vi "IV(H)_2devices_DC_vector_magnet_angle+temperature_sweep_BF_LD-400_K6221_K2182A_PK.vi"() -> ()   [LabVIEW 2016]
uses:
  <vilib>/Math Plots/2D Math Plots/2D Compass/2D Compass XCtrl/2D Compass.xctl
  <vilib>/Math Plots/2D Math Plots/2D Compass/2D Compass Datatype/2D Compass Datatype.lvclass
  <vilib>/Math Plots/2D Math Plots/2D Compass/2D Compass Datatype/Public/Plot Helper (Vector).vi
  Labview Drivers/Keithley 622x LV 2009/Keithley 622x.lvlib
  Labview Drivers/lake_shore_372/Lake Shore 372/Lake Shore 372.lvlib
panel:
  out "Still temperature (K)":dbl=0.747234 min=0.0 max=1000.0 step=1e-05 format="%^.5e"
  out "Still Output (%)":dbl=13.69 min=0.0 max=100.0 step=1e-05 format="%^.5e"
  out "Magnet temperature (K)":dbl=3.7122 min=0.0 max=1000.0 step=1e-05 format="%.5f"
  in  "From 5":dbl[](array[numeric])=[0.0] min=-3000.0 max=3000.0 format="%#.5f"
  in  "To 5":dbl[](array[numeric])=[0.0] min=-3000.0 max=3000.0 format="%#.5g"
  in  "Step 5":dbl[](array[numeric])=[0.001] min=-3000.0 max=3000.0 format="%.5e"
  in  "Still Heater Output (%)":dbl=13.69
  in  "Heater Range (0: Off)":u16(ring)=6 items=["Off", "31.6 uA", "100 uA", "316 uA", "1.00 mA", "3.16 mA", "10.0 mA", "31.6 mA", "100 mA"]
  in  "Output (0: sample heater)":u16(ring) items=["sample heater", "output 1 (warm-up heater) ", "output 2 (analog/still)"]
  in  "Rate(D) (0)":dbl min=0.0 max=2500.0 step=1.0 format="%.6f"
  in  "Reset(I) (20)":dbl=20.0 min=0.0 max=10000.0 step=1.0 format="%.6f"
  in  "Gain(P) (10.000)":dbl=10.0 min=0.001 max=1000.0 step=0.001 format="%.6f"
  out "Set Temperature (K)":dbl=0.9999999999999999 format="%#_13g"
  out "Delay timer (s)":i32=600
  in  "T settling delay (s)":i32=60
  out "Heater Output (%)":dbl=7.0 min=0.0 max=100.0 step=1e-05 format="%^.5e"
  out "Current Temperature (K)":dbl=1.00279 format="%#_13g"
  out "data 2":dbl[](array[numeric])=[0.0, 0.1539956170131437, 179.99925141305565, -5.8e-05, -0.000894677769, 15.42547877586207, 62218.001]
  out "File path 2":path=path "D:/Malli/GeTe/VNM519/027_VNM519_Dev1_DC_IV_baseT_OOP-Y-axis(250_to_-250mT)_1mT_steps_I16-19_V17-18_(K6221_12- K2182_4).dat"
  in  "Measure two devices?":bool
  out "2D Compass":refnum<class "2D Plot Datatype.lvclass">[](xcontrol)
  in  "Number Averaging":i32=1
  in  "Tab Control":enum32{"Device 1", "Device 2"}(tab)
  out "V vs I":cluster{dbl, "Field Reading":dbl}[](graph)=[{0.0, "Field Reading"=-1.52268497e-07}, {2e-07, "Field Reading"=-7.97594228e-08}, {4e-07, "Field Reading"=-2.74494669e-08}, {6e-07, "Field Reading"=2.5999633e-07}, {8e-07, "Field Reading"=6.6863549e-07}, {1e-06, "Field Reading"=9.26042323e-07}, {1.2e-06, "Field Reading"=1.14823021e-06}, {1.4e-06, "Field Reading"=1.4843606e-06}, {1.6e-06, "Field Reading"=1.76714547e-06}, {1.8e-06, "Field Reading"=1.96654487e-06}, {2e-06, "Field Reading"=2.31562332e-06}, {2.2e-06, "Field Reading"=2.42801356e-06}, {2.4e-06, "Field Reading"=2.6657392e-06}, {2.6e-06, "Field Reading"=3.04123176e-06}, {2.8e-06, "Field Reading"=3.30122805e-06}, {3e-06, "Field Reading"=3.42190359e-06}, {3.2e-06, "Field Reading"=3.80050368e-06}, {3.4e-06, "Field Reading"=3.8305433e-06}, {3.6e-06, "Field Reading"=4.18790866e-06}, {3.8e-06, "Field Reading"=4.36969886e-06}, {4e-06, "Field Reading"=4.7099712e-06}, {4.2e-06, "Field Reading"=5.08080239e-06}, {4.4e-06, "Field Reading"=5.22633809e-06}, {4.6e-06, "Field Reading"=5.43764972e-06}, {4.8e-06, "Field Reading"=5.58784671e-06}, {5e-06, "Field Reading"=5.92760266e-06}, {5.2e-06, "Field Reading"=6.16066695e-06}, {5.4e-06, "Field Reading"=6.52631866e-06}, {5.6e-06, "Field Reading"=6.60711428e-06}, {5.8e-06, "Field Reading"=6.8862735e-06}, {6e-06, "Field Reading"=7.20945277e-06}, {6.2e-06, "Field Reading"=7.31976981e-06}, {6.4e-06, "Field Reading"=7.68645747e-06}, {6.6e-06, "Field Reading"=7.9987682e-06}, {6.8e-06, "Field Reading"=8.25462103e-06}, {7e-06, "Field Reading"=8.2913934e-06}, {7.2e-06, "Field Reading"=8.71400919e-06}, {7.4e-06, "Field Reading"=8.98850694e-06}, {7.6e-06, "Field Reading"=9.18531665e-06}, {7.8e-06, "Field Reading"=9.47948819e-06}, {8e-06, "Field Reading"=9.61984449e-06}, {8.2e-06, "Field Reading"=9.91195133e-06}, {8.4e-06, "Field Reading"=1.00347079e-05}, {8.6e-06, "Field Reading"=1.03490855e-05}, {8.8e-06, "Field Reading"=1.06489614e-05}, {9e-06, "Field Reading"=1.08991132e-05}, {9.2e-06, "Field Reading"=1.1134249e-05}, {9.4e-06, "Field Reading"=1.13165569e-05}, {9.6e-06, "Field Reading"=1.15257967e-05}, {9.8e-06, "Field Reading"=1.18443188e-05}, {1e-05, "Field Reading"=1.21214061e-05}, {1.02e-05, "Field Reading"=1.23254667e-05}, {1.04e-05, "Field Reading"=1.26320829e-05}, {1.06e-05, "Field Reading"=1.27895307e-05}, {1.08e-05, "Field Reading"=1.30749049e-05}, {1.1e-05, "Field Reading"=1.32494289e-05}, {1.12e-05, "Field Reading"=1.34664374e-05}, {1.14e-05, "Field Reading"=1.3915992e-05}, {1.16e-05, "Field Reading"=1.40470318e-05}, {1.18e-05, "Field Reading"=1.43101353e-05}, {1.2e-05, "Field Reading"=1.45571832e-05}, {1.22e-05, "Field Reading"=1.46328053e-05}, {1.24e-05, "Field Reading"=1.50393728e-05}, {1.26e-05, "Field Reading"=1.51921593e-05}, {1.28e-05, "Field Reading"=1.54972138e-05}, {1.3e-05, "Field Reading"=1.57333855e-05}, {1.32e-05, "Field Reading"=1.59866486e-05}, {1.34e-05, "Field Reading"=1.6305696e-05}, {1.36e-05, "Field Reading"=1.64346582e-05}, {1.38e-05, "Field Reading"=1.66801526e-05}, {1.4e-05, "Field Reading"=1.69613835e-05}, {1.42e-05, "Field Reading"=1.71208941e-05}, {1.44e-05, "Field Reading"=1.74218058e-05}, {1.46e-05, "Field Reading"=1.76522803e-05}, {1.48e-05, "Field Reading"=1.80106844e-05}, {1.5e-05, "Field Reading"=1.80904442e-05}, {1.52e-05, "Field Reading"=1.83623524e-05}, {1.54e-05, "Field Reading"=1.86627412e-05}, {1.56e-05, "Field Reading"=1.88631763e-05}, {1.58e-05, "Field Reading"=1.90320183e-05}, {1.6e-05, "Field Reading"=1.93800576e-05}, {1.62e-05, "Field Reading"=1.9578939e-05}, {1.64e-05, "Field Reading"=1.97788562e-05}, {1.66e-05, "Field Reading"=2.00880632e-05}, {1.68e-05, "Field Reading"=2.0350131e-05}, {1.7e-05, "Field Reading"=2.05593708e-05}, {1.72e-05, "Field Reading"=2.0896531e-05}, {1.74e-05, "Field Reading"=2.10658909e-05}, {1.76e-05, "Field Reading"=2.11917455e-05}, {1.78e-05, "Field Reading"=2.15387632e-05}, {1.8e-05, "Field Reading"=2.17775246e-05}, {1.82e-05, "Field Reading"=2.19841749e-05}, {1.84e-05, "Field Reading"=2.22824971e-05}, {1.86e-05, "Field Reading"=2.24321761e-05}, {1.88e-05, "Field Reading"=2.27020127e-05}, {1.9e-05, "Field Reading"=2.29822077e-05}, {1.92e-05, "Field Reading"=2.32157907e-05}, {1.94e-05, "Field Reading"=2.3448855e-05}, {1.96e-05, "Field Reading"=2.36135537e-05}, {1.98e-05, "Field Reading"=2.38725181e-05}, {2e-05, "Field Reading"=2.41837884e-05}, {2.02e-05, "Field Reading"=2.43945821e-05}, {2.04e-05, "Field Reading"=2.46193413e-05}, {2.06e-05, "Field Reading"=2.49093766e-05}, {2.08e-05, "Field Reading"=2.51222418e-05}, {2.1e-05, "Field Reading"=2.52900611e-05}, {2.12e-05, "Field Reading"=2.55407347e-05}, {2.14e-05, "Field Reading"=2.58758293e-05}, {2.16e-05, "Field Reading"=2.60860873e-05}, {2.18e-05, "Field Reading"=2.6178795e-05}, {2.2e-05, "Field Reading"=2.6620063e-05}, {2.22e-05, "Field Reading"=2.67676686e-05}, {2.24e-05, "Field Reading"=2.69230447e-05}, {2.26e-05, "Field Reading"=2.72975009e-05}, {2.28e-05, "Field Reading"=2.7582357e-05}, {2.3e-05, "Field Reading"=2.77507011e-05}, {2.32e-05, "Field Reading"=2.80096614e-05}, {2.34e-05, "Field Reading"=2.81696988e-05}, {2.36e-05, "Field Reading"=2.85907685e-05}, {2.38e-05, "Field Reading"=2.87735944e-05}, {2.4e-05, "Field Reading"=2.90294472e-05}, {2.42e-05, "Field Reading"=2.9178615e-05}, {2.44e-05, "Field Reading"=2.96002024e-05}, {2.46e-05, "Field Reading"=2.9786136e-05}, {2.48e-05, "Field Reading"=2.99565396e-05}, {2.6e-05, "Field Reading"=3.14186299e-05}, {2.7e-05, "Field Reading"=3.26751057e-05}, {2.8e-05, "Field Reading"=3.38378258e-05}, {2.9e-05, "Field Reading"=3.52035824e-05}, {3e-05, "Field Reading"=3.63435256e-05}, {3e-05, "Field Reading"=3.63673343e-05}, {1.501e-05, "Field Reading"=1.79573366e-05}, {2e-08, "Field Reading"=-3.87921991e-07}, {0.0, "Field Reading"=-3.45452353e-07}, {-2e-07, "Field Reading"=-3.83778479e-07}, {-4e-07, "Field Reading"=-4.92023888e-07}, {-6e-07, "Field Reading"=-7.5460964e-07}, {-8e-07, "Field Reading"=-1.24196958e-06}, {-1e-06, "Field Reading"=-1.538736e-06}, {-1.2e-06, "Field Reading"=-1.68893191e-06}, {-1.4e-06, "Field Reading"=-2.02972104e-06}, {-1.6e-06, "Field Reading"=-2.24103112e-06}, {-1.8e-06, "Field Reading"=-2.59114291e-06}, {-2e-06, "Field Reading"=-2.7993462e-06}, {-2.2e-06, "Field Reading"=-2.92209253e-06}, {-2.4e-06, "Field Reading"=-3.30068989e-06}, {-2.6e-06, "Field Reading"=-3.44466872e-06}, {-2.8e-06, "Field Reading"=-3.70673454e-06}, {-3e-06, "Field Reading"=-3.97190785e-06}, {-3.2e-06, "Field Reading"=-4.17493005e-06}, {-3.4e-06, "Field Reading"=-4.41472537e-06}, {-3.6e-06, "Field Reading"=-4.66177152e-06}, {-3.8e-06, "Field Reading"=-4.9191763e-06}, {-4e-06, "Field Reading"=-5.20920954e-06}, {-4.2e-06, "Field Reading"=-5.55465984e-06}, {-4.4e-06, "Field Reading"=-5.66652605e-06}, {-4.6e-06, "Field Reading"=-5.96691739e-06}, {-4.8e-06, "Field Reading"=-6.19013923e-06}, {-5e-06, "Field Reading"=-6.40818191e-06}, {-5.2e-06, "Field Reading"=-6.672842e-06}, {-5.4e-06, "Field Reading"=-6.9483736e-06}, {-5.6e-06, "Field Reading"=-7.18713312e-06}, {-5.8e-06, "Field Reading"=-7.36218605e-06}, {-6e-06, "Field Reading"=-7.68329416e-06}, {-6.2e-06, "Field Reading"=-7.86922612e-06}, {-6.4e-06, "Field Reading"=-8.26853861e-06}, {-6.6e-06, "Field Reading"=-8.30634649e-06}, {-6.8e-06, "Field Reading"=-8.59586168e-06}, {-7e-06, "Field Reading"=-9.00657456e-06}, {-7.2e-06, "Field Reading"=-9.14951953e-06}, {-7.4e-06, "Field Reading"=-9.39708366e-06}, {-7.6e-06, "Field Reading"=-9.56643916e-06}, {-7.8e-06, "Field Reading"=-9.81970027e-06}, {-8e-06, "Field Reading"=-1.00263489e-05}, {-8.2e-06, "Field Reading"=-1.02837565e-05}, {-8.4e-06, "Field Reading"=-1.06437086e-05}, {-8.6e-06, "Field Reading"=-1.07623114e-05}, {-8.8e-06, "Field Reading"=-1.09855426e-05}, {-9e-06, "Field Reading"=-1.11694032e-05}, {-9.2e-06, "Field Reading"=-1.15034596e-05}, {-9.4e-06, "Field Reading"=-1.17209848e-05}, {-9.6e-06, "Field Reading"=-1.19462748e-05}, {-9.8e-06, "Field Reading"=-1.21871062e-05}, {-1e-05, "Field Reading"=-1.24362242e-05}, {-1.02e-05, "Field Reading"=-1.26667036e-05}, {-1.04e-05, "Field Reading"=-1.30364964e-05}, {-1.06e-05, "Field Reading"=-1.32317511e-05}, {-1.08e-05, "Field Reading"=-1.35373222e-05}, {-1.1e-05, "Field Reading"=-1.37237724e-05}, {-1.12e-05, "Field Reading"=-1.40371123e-05}, {-1.14e-05, "Field Reading"=-1.42893266e-05}, {-1.16e-05, "Field Reading"=-1.43830695e-05}, {-1.18e-05, "Field Reading"=-1.46358129e-05}, {-1.2e-05, "Field Reading"=-1.50543024e-05}, {-1.22e-05, "Field Reading"=-1.51656546e-05}, {-1.24e-05, "Field Reading"=-1.54468836e-05}, {-1.26e-05, "Field Reading"=-1.56442061e-05}, {-1.28e-05, "Field Reading"=-1.580735e-05}, {-1.3e-05, "Field Reading"=-1.61113673e-05}, {-1.32e-05, "Field Reading"=-1.62418839e-05}, {-1.34e-05, "Field Reading"=-1.6634983e-05}, {-1.36e-05, "Field Reading"=-1.68178077e-05}, {-1.38e-05, "Field Reading"=-1.69198374e-05}, {-1.4e-05, "Field Reading"=-1.7212986e-05}, {-1.42e-05, "Field Reading"=-1.74341367e-05}, {-1.44e-05, "Field Reading"=-1.77231346e-05}, {-1.46e-05, "Field Reading"=-1.78510457e-05}, {-1.48e-05, "Field Reading"=-1.81830304e-05}, {-1.5e-05, "Field Reading"=-1.83668909e-05}, {-1.52e-05, "Field Reading"=-1.86812606e-05}, {-1.54e-05, "Field Reading"=-1.87755215e-05}, {-1.56e-05, "Field Reading"=-1.91867473e-05}, {-1.58e-05, "Field Reading"=-1.92447572e-05}, {-1.6e-05, "Field Reading"=-1.95373802e-05}, {-1.62e-05, "Field Reading"=-1.98776515e-05}, {-1.64e-05, "Field Reading"=-2.01619878e-05}, {-1.66e-05, "Field Reading"=-2.03448124e-05}, {-1.68e-05, "Field Reading"=-2.05985916e-05}, {-1.7e-05, "Field Reading"=-2.09740769e-05}, {-1.72e-05, "Field Reading"=-2.10243148e-05}, {-1.74e-05, "Field Reading"=-2.14578111e-05}, {-1.76e-05, "Field Reading"=-2.17752926e-05}, {-1.78e-05, "Field Reading"=-2.20503063e-05}, {-1.8e-05, "Field Reading"=-2.21507822e-05}, {-1.82e-05, "Field Reading"=-2.23900597e-05}, {-1.84e-05, "Field Reading"=-2.26723233e-05}, {-1.86e-05, "Field Reading"=-2.28976171e-05}, {-1.88e-05, "Field Reading"=-2.31016762e-05}, {-1.9e-05, "Field Reading"=-2.34289957e-05}, {-1.92e-05, "Field Reading"=-2.37117782e-05}, {-1.94e-05, "Field Reading"=-2.40458343e-05}, {-1.96e-05, "Field Reading"=-2.40541191e-05}, {-1.98e-05, "Field Reading"=-2.44544686e-05}, {-2e-05, "Field Reading"=-2.46621531e-05}, {-2.02e-05, "Field Reading"=-2.49703066e-05}, {-2.04e-05, "Field Reading"=-2.5097714e-05}, {-2.06e-05, "Field Reading"=-2.54835617e-05}, {-2.08e-05, "Field Reading"=-2.55648796e-05}, {-2.1e-05, "Field Reading"=-2.58497336e-05}, {-2.12e-05, "Field Reading"=-2.60413627e-05}, {-2.14e-05, "Field Reading"=-2.64365387e-05}, {-2.16e-05, "Field Reading"=-2.67032657e-05}, {-2.18e-05, "Field Reading"=-2.68964486e-05}, {-2.2e-05, "Field Reading"=-2.71341792e-05}, {-2.22e-05, "Field Reading"=-2.72719451e-05}, {-2.24e-05, "Field Reading"=-2.75303855e-05}, {-2.26e-05, "Field Reading"=-2.79266128e-05}, {-2.28e-05, "Field Reading"=-2.81301542e-05}, {-2.3e-05, "Field Reading"=-2.83901486e-05}, {-2.32e-05, "Field Reading"=-2.84232953e-05}, {-2.34e-05, "Field Reading"=-2.87630526e-05}, {-2.36e-05, "Field Reading"=-2.91333634e-05}, {-2.38e-05, "Field Reading"=-2.9317224e-05}, {-2.4e-05, "Field Reading"=-2.96481828e-05}, {-2.42e-05, "Field Reading"=-2.98304898e-05}, {-2.44e-05, "Field Reading"=-2.99692916e-05}, {-2.46e-05, "Field Reading"=-3.02660647e-05}, {-2.48e-05, "Field Reading"=-3.04944663e-05}, {-2.6e-05, "Field Reading"=-3.20653099e-05}, {-2.7e-05, "Field Reading"=-3.32523697e-05}, {-2.8e-05, "Field Reading"=-3.44534201e-05}, {-2.9e-05, "Field Reading"=-3.56938321e-05}, {-3e-05, "Field Reading"=-3.69958442e-05}, {-3e-05, "Field Reading"=-3.70222579e-05}, {-1.501e-05, "Field Reading"=-1.84243803e-05}, {-2e-08, "Field Reading"=-2.59477872e-07}]
  in  "File name 1":string="011_31-05-2022_DevB4_DC_IV(H)_baseT_[5_to-5mT]_30uT_steps_(0_deg)_I_10-36_V_12-37_100nA_steps"
  in  "From 3":dbl[](array[numeric])=[0.0, 2e-05, 0.0, -2e-05] min=-3000.0 max=3000.0 format="%.1e"
  in  "To 3":dbl[](array[numeric])=[2e-05, 0.0, -2e-05, 0.0] min=-3000.0 max=3000.0 format="%.1e"
  in  "Step 3":dbl[](array[numeric])=[2e-08, 9.99e-06, 2e-08, 9.99e-06] min=-3000.0 max=3000.0 format="%.1e"
  in  "Current source K6221 VISA Device 1":refnum<visa-resource-name>="GPIB0::13::INSTR"
  in  "Nanovoltmeter 2182a VISA Device1":refnum<visa-resource-name>="GPIB0::7::INSTR"
  in  "wait (ms)":u32=50
  in  "Set Compliance voltage (V)":dbl=2.0 min=0.0 step=0.1 format="%_3f"
  out "Resistance (ohm)":dbl=12.9738936 format="%#_13g"
  out "Time (s)":dbl=151861.951 format="%#_13g"
  out "Iset (A)":dbl=-2e-08
  out "Vmeas (V)":dbl=-2.59477872e-07
  in  "File name 2":string="040_31-05-2023_DevB3_DC_IV(A)_baseT_12mT_(0-360deg)_5deg_steps_I_10-38_V_12-31_"
  in  "Current source K6221 VISA Device 2":refnum<visa-resource-name>="GPIB0::13::INSTR"
  in  "Nanovoltmeter 2182a VISA Device 2":refnum<visa-resource-name>="GPIB0::7::INSTR"
  in  "Set Compliance voltage (V) 2":dbl=2.0 min=0.0 step=0.1 format="%_3f"
  in  "wait (ms) 2":u32=50
  in  "To 4":dbl[](array[numeric])=[1e-05, 3e-05, -1e-05, -0.0001, 0.0] min=-3000.0 max=3000.0 format="%.1e"
  in  "From 4":dbl[](array[numeric])=[0.0, 1.1e-05, 3e-05, 0.0, -0.0001] min=-3000.0 max=3000.0 format="%.1e"
  in  "Step 4":dbl[](array[numeric])=[2e-07, 1e-06, 0.0, 5e-07, 9.9e-05] min=-3000.0 max=3000.0 format="%.1e"
  out "V vs I 2":cluster{dbl, "Field Reading":dbl}[](graph)=[{0.0, "Field Reading"=1.05982577e-07}, {5e-07, "Field Reading"=1.23902621e-07}, {1e-06, "Field Reading"=4.09598972e-08}, {1.5e-06, "Field Reading"=7.78233302e-08}, {2e-06, "Field Reading"=7.52633791e-08}, {2.5e-06, "Field Reading"=9.9839001e-08}, {3e-06, "Field Reading"=6.70715052e-08}, {3.5e-06, "Field Reading"=6.34878296e-08}, {4e-06, "Field Reading"=1.95069789e-07}, {4.5e-06, "Field Reading"=1.48733775e-06}, {5e-06, "Field Reading"=3.68225755e-06}, {5.5e-06, "Field Reading"=7.0056209e-06}, {6e-06, "Field Reading"=1.131355e-05}, {6.5e-06, "Field Reading"=1.67191983e-05}, {7e-06, "Field Reading"=2.2852904e-05}, {7.5e-06, "Field Reading"=2.94079847e-05}, {8e-06, "Field Reading"=3.63951874e-05}, {8.5e-06, "Field Reading"=4.35057808e-05}, {9e-06, "Field Reading"=5.09056291e-05}, {9.5e-06, "Field Reading"=5.82773365e-05}, {1e-05, "Field Reading"=6.58016184e-05}, {1.05e-05, "Field Reading"=7.33770992e-05}, {1.1e-05, "Field Reading"=8.09648681e-05}, {1.15e-05, "Field Reading"=8.87364392e-05}, {1.2e-05, "Field Reading"=9.64209746e-05}, {1.25e-05, "Field Reading"=0.000104230437}, {1.3e-05, "Field Reading"=0.000112046003}, {1.35e-05, "Field Reading"=0.000119815015}, {1.4e-05, "Field Reading"=0.000127742783}, {1.45e-05, "Field Reading"=0.000135573235}, {1.5e-05, "Field Reading"=0.000143516327}, {1.55e-05, "Field Reading"=0.000151494156}, {1.6e-05, "Field Reading"=0.000159501242}, {1.65e-05, "Field Reading"=0.000167343466}, {1.7e-05, "Field Reading"=0.000175483152}, {1.75e-05, "Field Reading"=0.000183456446}, {1.8e-05, "Field Reading"=0.000191661699}, {1.85e-05, "Field Reading"=0.000199612466}, {1.9e-05, "Field Reading"=0.000207719848}, {1.95e-05, "Field Reading"=0.000215802195}, {2e-05, "Field Reading"=0.00022388403}, {2.05e-05, "Field Reading"=0.000232062763}, {2.1e-05, "Field Reading"=0.000240102107}, {2.15e-05, "Field Reading"=0.000247269011}, {2.2e-05, "Field Reading"=0.000255929973}, {2.25e-05, "Field Reading"=0.000264142372}, {2.3e-05, "Field Reading"=0.000272170452}, {2.35e-05, "Field Reading"=0.000280406012}, {2.4e-05, "Field Reading"=0.000288539055}, {2.45e-05, "Field Reading"=0.000296639977}, {2.5e-05, "Field Reading"=0.000304956829}, {2.55e-05, "Field Reading"=0.000312984916}, {2.6e-05, "Field Reading"=0.000321277684}, {2.65e-05, "Field Reading"=0.000329427113}, {2.7e-05, "Field Reading"=0.00033774076}, {2.75e-05, "Field Reading"=0.000346032008}, {2.8e-05, "Field Reading"=0.000354167609}, {2.85e-05, "Field Reading"=0.000362498087}, {2.9e-05, "Field Reading"=0.000370754002}, {2.95e-05, "Field Reading"=0.000379070387}, {3e-05, "Field Reading"=0.000387405662}, {3.05e-05, "Field Reading"=0.000395624202}, {3.1e-05, "Field Reading"=0.000403926088}, {3.15e-05, "Field Reading"=0.00041243339}, {3.2e-05, "Field Reading"=0.000420845302}, {3.25e-05, "Field Reading"=0.000429363875}, {3.3e-05, "Field Reading"=0.000437565523}, {3.35e-05, "Field Reading"=0.000446109155}, {3.4e-05, "Field Reading"=0.000454533008}, {3.45e-05, "Field Reading"=0.000463127356}, {3.5e-05, "Field Reading"=0.000471630056}, {3.55e-05, "Field Reading"=0.000479936662}, {3.6e-05, "Field Reading"=0.000488525981}, {3.65e-05, "Field Reading"=0.000497198664}, {3.7e-05, "Field Reading"=0.000505853053}, {3.75e-05, "Field Reading"=0.000514436643}, {3.8e-05, "Field Reading"=0.000522915273}, {3.85e-05, "Field Reading"=0.000531648928}, {3.9e-05, "Field Reading"=0.000540244293}, {3.95e-05, "Field Reading"=0.000548950249}, {4e-05, "Field Reading"=0.000557677924}, {4.05e-05, "Field Reading"=0.000566248716}, {4.1e-05, "Field Reading"=0.000574937679}, {4.15e-05, "Field Reading"=0.000583695347}, {4.2e-05, "Field Reading"=0.000592494999}, {4.25e-05, "Field Reading"=0.000601192661}, {4.3e-05, "Field Reading"=0.000609976951}, {4.35e-05, "Field Reading"=0.000618619419}, {4.4e-05, "Field Reading"=0.000627518275}, {4.45e-05, "Field Reading"=0.000636379362}, {4.5e-05, "Field Reading"=0.000644912509}, {4.55e-05, "Field Reading"=0.00065393999}, {4.6e-05, "Field Reading"=0.000662870466}, {4.65e-05, "Field Reading"=0.000671738209}, {4.7e-05, "Field Reading"=0.000680896763}, {4.75e-05, "Field Reading"=0.000689596876}, {4.8e-05, "Field Reading"=0.000698582898}, {4.85e-05, "Field Reading"=0.000707876118}, {4.9e-05, "Field Reading"=0.00071700519}, {4.95e-05, "Field Reading"=0.00072625694}, {5e-05, "Field Reading"=0.000735252693}, {5.05e-05, "Field Reading"=0.000744563505}, {5.1e-05, "Field Reading"=0.000753877714}, {5.15e-05, "Field Reading"=0.000763235462}, {5.2e-05, "Field Reading"=0.000772666405}, {5.25e-05, "Field Reading"=0.000781939653}, {5.3e-05, "Field Reading"=0.00079146705}, {5.35e-05, "Field Reading"=0.000801081283}, {5.4e-05, "Field Reading"=0.000810671964}, {5.45e-05, "Field Reading"=0.000820330099}, {5.5e-05, "Field Reading"=0.000830001161}, {5.55e-05, "Field Reading"=0.000839830429}, {5.6e-05, "Field Reading"=0.000849894446}, {5.65e-05, "Field Reading"=0.000859963842}, {5.7e-05, "Field Reading"=0.00087027569}, {5.75e-05, "Field Reading"=0.000880684023}, {5.8e-05, "Field Reading"=0.000891300225}, {5.85e-05, "Field Reading"=0.000901884572}, {5.9e-05, "Field Reading"=0.00091264413}, {5.95e-05, "Field Reading"=0.000923292586}, {6e-05, "Field Reading"=0.000933904184}, {6.05e-05, "Field Reading"=0.000944740541}, {6.1e-05, "Field Reading"=0.000955724863}, {6.15e-05, "Field Reading"=0.000966541693}, {6.2e-05, "Field Reading"=0.000977790203}, {6.25e-05, "Field Reading"=0.0009887668}, {6.3e-05, "Field Reading"=0.00100003886}, {6.35e-05, "Field Reading"=0.00101126331}, {6.4e-05, "Field Reading"=0.00102284095}, {6.45e-05, "Field Reading"=0.00103437413}, {6.5e-05, "Field Reading"=0.00104578697}, {6.55e-05, "Field Reading"=0.00105781627}, {6.6e-05, "Field Reading"=0.00106970781}, {6.65e-05, "Field Reading"=0.00108158658}, {6.7e-05, "Field Reading"=0.00109345152}, {6.75e-05, "Field Reading"=0.00110520407}, {6.8e-05, "Field Reading"=0.00111705365}, {6.85e-05, "Field Reading"=0.00112896007}, {6.9e-05, "Field Reading"=0.00114097245}, {6.95e-05, "Field Reading"=0.00115300225}, {7e-05, "Field Reading"=0.00116490713}, {7.05e-05, "Field Reading"=0.00117701585}, {7.1e-05, "Field Reading"=0.0011890902}, {7.15e-05, "Field Reading"=0.00120116737}, {7.2e-05, "Field Reading"=0.00121302054}, {7.25e-05, "Field Reading"=0.00122527818}, {7.3e-05, "Field Reading"=0.00123750597}, {7.35e-05, "Field Reading"=0.00124952144}, {7.4e-05, "Field Reading"=0.00126179393}, {7.45e-05, "Field Reading"=0.00127385138}, {7.5e-05, "Field Reading"=0.00128607011}, {7.55e-05, "Field Reading"=0.00129831901}, {7.6e-05, "Field Reading"=0.00131059815}, {7.65e-05, "Field Reading"=0.00132285322}, {7.7e-05, "Field Reading"=0.00133496366}, {7.75e-05, "Field Reading"=0.00134726123}, {7.8e-05, "Field Reading"=0.00135956111}, {7.85e-05, "Field Reading"=0.00137195033}, {7.9e-05, "Field Reading"=0.00138423407}, {7.95e-05, "Field Reading"=0.00139647286}, {8e-05, "Field Reading"=0.00140887898}, {8.05e-05, "Field Reading"=0.00142125669}, {8.1e-05, "Field Reading"=0.00143369762}, {8.15e-05, "Field Reading"=0.00144604179}, {8.2e-05, "Field Reading"=0.00145820055}, {8.25e-05, "Field Reading"=0.0014708299}, {8.3e-05, "Field Reading"=0.001483259}, {8.35e-05, "Field Reading"=0.00149571273}, {8.4e-05, "Field Reading"=0.00150827449}, {8.45e-05, "Field Reading"=0.00152058173}, {8.5e-05, "Field Reading"=0.00153315169}, {8.55e-05, "Field Reading"=0.00154567403}, {8.6e-05, "Field Reading"=0.00155821094}, {8.65e-05, "Field Reading"=0.00157085359}, {8.7e-05, "Field Reading"=0.00158327521}, {8.75e-05, "Field Reading"=0.00159591991}, {8.8e-05, "Field Reading"=0.00160856665}, {8.85e-05, "Field Reading"=0.00162121374}, {8.9e-05, "Field Reading"=0.00163385997}, {8.95e-05, "Field Reading"=0.00164634288}, {9e-05, "Field Reading"=0.00165906267}, {9.05e-05, "Field Reading"=0.00167177904}, {9.1e-05, "Field Reading"=0.00168450438}, {9.15e-05, "Field Reading"=0.00169730779}, {9.2e-05, "Field Reading"=0.00170982705}, {9.25e-05, "Field Reading"=0.00172262613}, {9.3e-05, "Field Reading"=0.00173539114}, {9.35e-05, "Field Reading"=0.00174822988}, {9.4e-05, "Field Reading"=0.00176107221}, {9.45e-05, "Field Reading"=0.00177372408}, {9.5e-05, "Field Reading"=0.00178659463}, {9.55e-05, "Field Reading"=0.00179942159}, {9.6e-05, "Field Reading"=0.00181213335}, {9.65e-05, "Field Reading"=0.00182507038}, {9.7e-05, "Field Reading"=0.00183795264}, {9.75e-05, "Field Reading"=0.00185079437}, {9.8e-05, "Field Reading"=0.0018638159}, {9.85e-05, "Field Reading"=0.00187644421}, {9.9e-05, "Field Reading"=0.0018893681}, {9.95e-05, "Field Reading"=0.001902598}, {0.0001, "Field Reading"=0.00191566643}, {0.0001, "Field Reading"=0.00191578214}, {1e-06, "Field Reading"=1.04959382e-07}, {0.0, "Field Reading"=6.2978119e-08}, {-5e-07, "Field Reading"=7.37299411e-08}, {-1e-06, "Field Reading"=7.32183306e-08}, {-1.5e-06, "Field Reading"=9.8305911e-08}, {-2e-06, "Field Reading"=9.8305911e-08}, {-2.5e-06, "Field Reading"=-9.212857e-09}, {-3e-06, "Field Reading"=7.52657514e-08}, {-3.5e-06, "Field Reading"=-2.29881222e-07}, {-4e-06, "Field Reading"=-9.66638942e-07}, {-4.5e-06, "Field Reading"=-2.71867509e-06}, {-5e-06, "Field Reading"=-5.44042382e-06}, {-5.5e-06, "Field Reading"=-9.24299578e-06}, {-6e-06, "Field Reading"=-1.39195329e-05}, {-6.5e-06, "Field Reading"=-1.93947706e-05}, {-7e-06, "Field Reading"=-2.53845658e-05}, {-7.5e-06, "Field Reading"=-3.17772987e-05}, {-8e-06, "Field Reading"=-3.85647725e-05}, {-8.5e-06, "Field Reading"=-4.54935603e-05}, {-9e-06, "Field Reading"=-5.25713378e-05}, {-9.5e-06, "Field Reading"=-5.9848778e-05}, {-1e-05, "Field Reading"=-6.72593486e-05}, {-1.05e-05, "Field Reading"=-7.46959979e-05}, {-1.1e-05, "Field Reading"=-8.22145956e-05}, {-1.15e-05, "Field Reading"=-8.98888387e-05}, {-1.2e-05, "Field Reading"=-9.7508345e-05}, {-1.25e-05, "Field Reading"=-0.000105279358}, {-1.3e-05, "Field Reading"=-0.000112994564}, {-1.35e-05, "Field Reading"=-0.000120810121}, {-1.4e-05, "Field Reading"=-0.000128620045}, {-1.45e-05, "Field Reading"=-0.00013646688}, {-1.5e-05, "Field Reading"=-0.000144369477}, {-1.55e-05, "Field Reading"=-0.000152356042}, {-1.6e-05, "Field Reading"=-0.00016028334}, {-1.65e-05, "Field Reading"=-0.000168222807}, {-1.7e-05, "Field Reading"=-0.000176283573}, {-1.75e-05, "Field Reading"=-0.000184271677}, {-1.8e-05, "Field Reading"=-0.000192294085}, {-1.85e-05, "Field Reading"=-0.000200345666}, {-1.9e-05, "Field Reading"=-0.00020833633}, {-1.95e-05, "Field Reading"=-0.000216423693}, {-2e-05, "Field Reading"=-0.000224573584}, {-2.05e-05, "Field Reading"=-0.000232658964}, {-2.1e-05, "Field Reading"=-0.000240789835}, {-2.15e-05, "Field Reading"=-0.00024942458}, {-2.2e-05, "Field Reading"=-0.000257524758}, {-2.25e-05, "Field Reading"=-0.000265682837}, {-2.3e-05, "Field Reading"=-0.000273921299}, {-2.35e-05, "Field Reading"=-0.000281918732}, {-2.4e-05, "Field Reading"=-0.000290019983}, {-2.45e-05, "Field Reading"=-0.000298346441}, {-2.5e-05, "Field Reading"=-0.000306562888}, {-2.55e-05, "Field Reading"=-0.000314745032}, {-2.6e-05, "Field Reading"=-0.000322866101}, {-2.65e-05, "Field Reading"=-0.000331147056}, {-2.7e-05, "Field Reading"=-0.000339239598}, {-2.75e-05, "Field Reading"=-0.000347604575}, {-2.8e-05, "Field Reading"=-0.000355902938}, {-2.85e-05, "Field Reading"=-0.000364053667}, {-2.9e-05, "Field Reading"=-0.000372274716}, {-2.95e-05, "Field Reading"=-0.000380721042}, {-3e-05, "Field Reading"=-0.000389052226}, {-3.05e-05, "Field Reading"=-0.000397248701}, {-3.1e-05, "Field Reading"=-0.000405627052}, {-3.15e-05, "Field Reading"=-0.000414022694}, {-3.2e-05, "Field Reading"=-0.000422452566}, {-3.25e-05, "Field Reading"=-0.000430871246}, {-3.3e-05, "Field Reading"=-0.000439115251}, {-3.35e-05, "Field Reading"=-0.000447710054}, {-3.4e-05, "Field Reading"=-0.000456261339}, {-3.45e-05, "Field Reading"=-0.000464751635}, {-3.5e-05, "Field Reading"=-0.000473286534}, {-3.55e-05, "Field Reading"=-0.00048171494}, {-3.6e-05, "Field Reading"=-0.000490283148}, {-3.65e-05, "Field Reading"=-0.000498827776}, {-3.7e-05, "Field Reading"=-0.000507439986}, {-3.75e-05, "Field Reading"=-0.000516045781}, {-3.8e-05, "Field Reading"=-0.0005246155}, {-3.85e-05, "Field Reading"=-0.000533221482}, {-3.9e-05, "Field Reading"=-0.000541909479}, {-3.95e-05, "Field Reading"=-0.000550577507}, {-4e-05, "Field Reading"=-0.000559311386}, {-4.05e-05, "Field Reading"=-0.000567846814}, {-4.1e-05, "Field Reading"=-0.00057664276}, {-4.15e-05, "Field Reading"=-0.000585338952}, {-4.2e-05, "Field Reading"=-0.000594088391}, {-4.25e-05, "Field Reading"=-0.00060273111}, {-4.3e-05, "Field Reading"=-0.000611546081}, {-4.35e-05, "Field Reading"=-0.00062030934}, {-4.4e-05, "Field Reading"=-0.000629159621}, {-4.45e-05, "Field Reading"=-0.0006379664}, {-4.5e-05, "Field Reading"=-0.000646666684}, {-4.55e-05, "Field Reading"=-0.000655509687}, {-4.6e-05, "Field Reading"=-0.000664396847}, {-4.65e-05, "Field Reading"=-0.000673287336}, {-4.7e-05, "Field Reading"=-0.000682299425}, {-4.75e-05, "Field Reading"=-0.000691233691}, {-4.8e-05, "Field Reading"=-0.000700295086}, {-4.85e-05, "Field Reading"=-0.00070939524}, {-4.9e-05, "Field Reading"=-0.000718437027}, {-4.95e-05, "Field Reading"=-0.000727632333}, {-5e-05, "Field Reading"=-0.000736695622}, {-5.05e-05, "Field Reading"=-0.000746025716}, {-5.1e-05, "Field Reading"=-0.000755243116}, {-5.15e-05, "Field Reading"=-0.000764786655}, {-5.2e-05, "Field Reading"=-0.000774240444}, {-5.25e-05, "Field Reading"=-0.000783658543}, {-5.3e-05, "Field Reading"=-0.000793342878}, {-5.35e-05, "Field Reading"=-0.000803049948}, {-5.4e-05, "Field Reading"=-0.000812865349}, {-5.45e-05, "Field Reading"=-0.000822671023}, {-5.5e-05, "Field Reading"=-0.000832792343}, {-5.55e-05, "Field Reading"=-0.000842879097}, {-5.6e-05, "Field Reading"=-0.000853268375}, {-5.65e-05, "Field Reading"=-0.000863553781}, {-5.7e-05, "Field Reading"=-0.00087382946}, {-5.75e-05, "Field Reading"=-0.000884019633}, {-5.8e-05, "Field Reading"=-0.000894677769}]
  out "Vmeas (V) 2":dbl=-0.000894677769
  out "Resistance (ohm) 2":dbl=15.42547877586207 format="%#_13g"
  out "Iset (A) 2":dbl=-5.8e-05
  out "Magnetic Field Vector Angle":dbl=284.9997059221995 format="%#_13g"
  out "Magnetic Field Vector magnitude (T)":dbl=0.11799861557435369 format="%#_13g"
  in  "From 2":dbl[](array[numeric])=[0.005] min=-3000.0 max=3000.0 format="%#.5f"
  in  "To 2":dbl[](array[numeric])=[-0.005] min=-3000.0 max=3000.0 format="%#.5g"
  in  "Step 2":dbl[](array[numeric])=[3e-05] min=-3000.0 max=3000.0 format="%.5e"
  in  "Wait time after each sweep(min)":dbl=0.1 format="%#_13g"
  out "Z-axis Magnetic Field (T)":string="-0.113978067\r\n"
  in  "Y-axis Field ramp rate (T/min)":string="0.0005"
  in  "Z-axis Field ramp rate (T/min)":string="0.0005"
  out "Z-axis (90 deg)":dbl(slide)=-0.113978067 scale=0.0..3.0
  out "Y-Axis (0deg)":dbl(slide)=0.030539704 scale=0.0..3.0
  out "Y-axis Magnetic Field (T)":string="0.030539704\r\n"
  in  "Magnet IP Address Z-axis":string="169.254.207.70"
  in  "Magnet IP Address Y-axis":string="169.254.67.34"
  in  "Magnetic field stabilization time (s)":dbl=1.0 format="%#_13g"
  in  "Step":dbl[](array[numeric])=[0.001] min=-3000.0 max=3000.0 format="%.4g"
  in  "To":dbl[](array[numeric])=[0.0] min=-3000.0 max=3000.0 format="%.4f"
  in  "From":dbl[](array[numeric])=[0.0] min=-3000.0 max=3000.0 format="%.4f"
  in  "Folder":path=path "D:/Pranava/Data/PtTe2/31-05-2022/001/Round8_IP/after warmup"
  out "data":dbl[](array[numeric])=[1.00279, 0.11799861557435369, 284.9997059221995, -2e-08, -2.59477872e-07, 12.9738936, 151861.951]
  out "File path 1":path=path "D:/Pranava/Data/PtTe2/31-05-2022/001/Round8_IP/after warmup/011_31-05-2022_DevB4_DC_IV(H)_baseT_[5_to-5mT]_30uT_steps_(0_deg)_I_10-36_V_12-37_100nA_steps.dat"
  # "11.5% corresponds to 7mW\n13.69% corresponds to 10mW\nSet to 0 if you want to use at 1K"
  # "[Must be less than 0.05]"
  # "It is important that there is enough time for the magnet to cool down after each sweep (Typically 15-20 min)"
  # "Configure Temperature (K)"
  # "Configure Field magnitude (T)"
  # "Configure Field Angle (deg)"
  # "Z-Axis: In-plane (90 deg)\nY-axis: Out-of-plane (0 deg)"
  # ".dat"
  # "Configure current sweep 1 (A)"
  # ".dat"
  # "Configure current sweep 2 (A)"
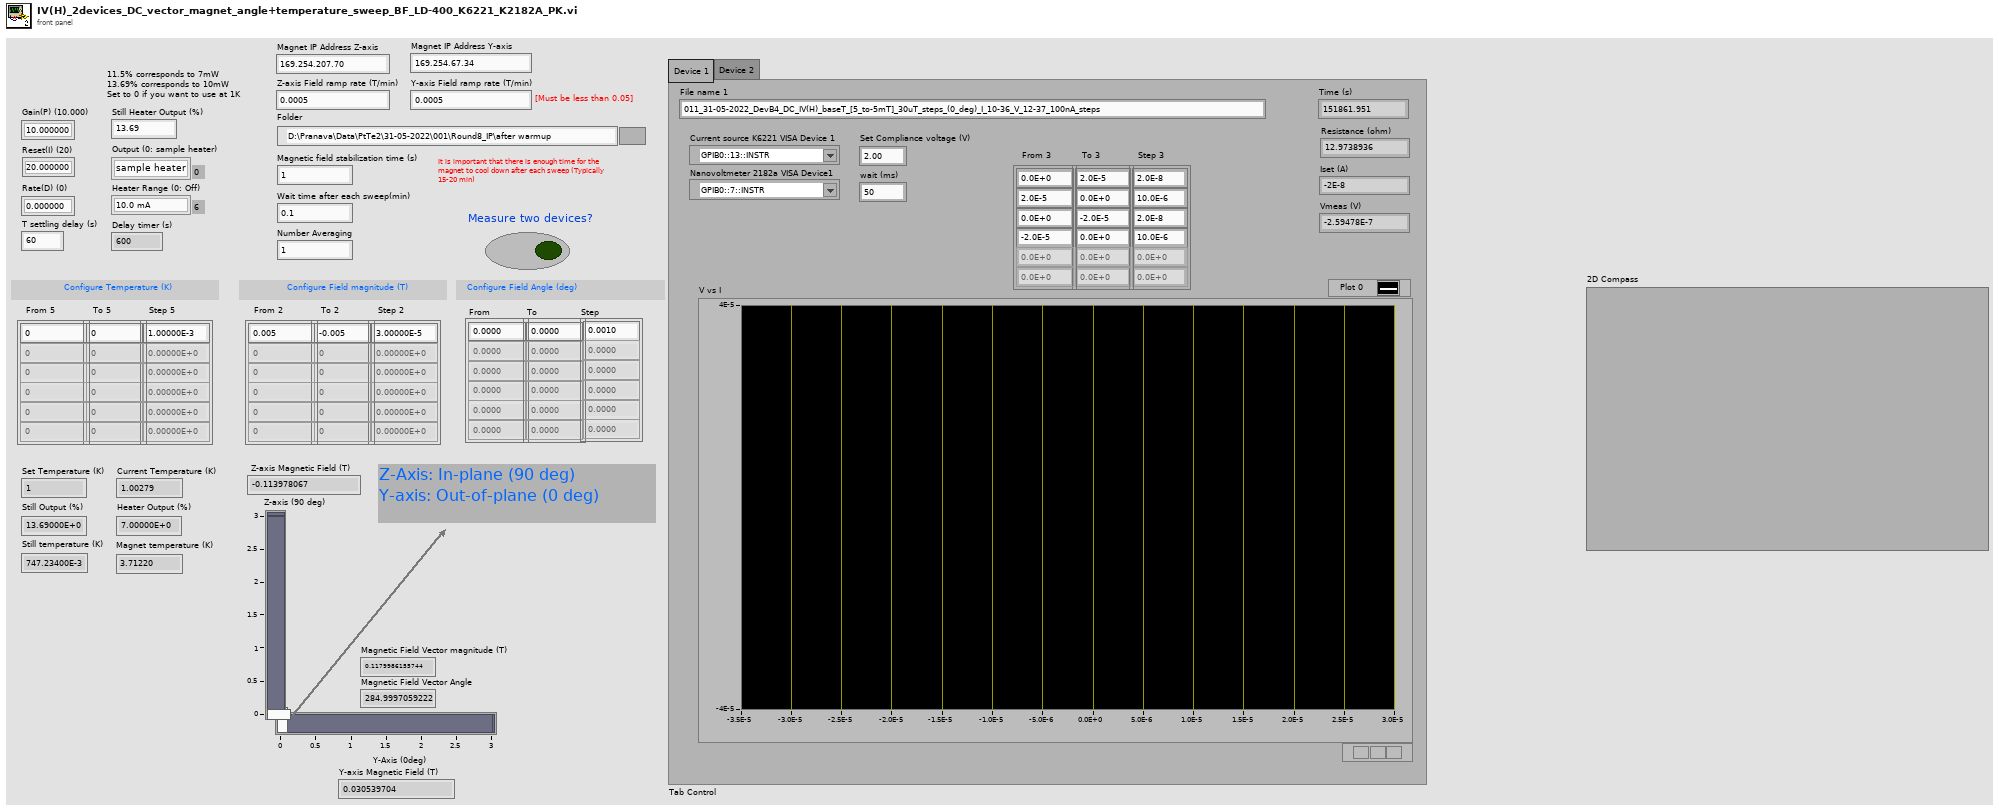
[diagram p1: front panel]
types:
  T1 = enum16{"open", "replace", "create", "open or create", "replace or create", "replace or create with confirmation"}
  T2 = typedef "Keithley 622x.lvlib/KE622x -- Current Level.ctl" = dbl
  T3 = cluster{"Average value":dbl, "Average value":dbl}
  T4 = cluster{"Average value":dbl, "Average value":dbl}[]
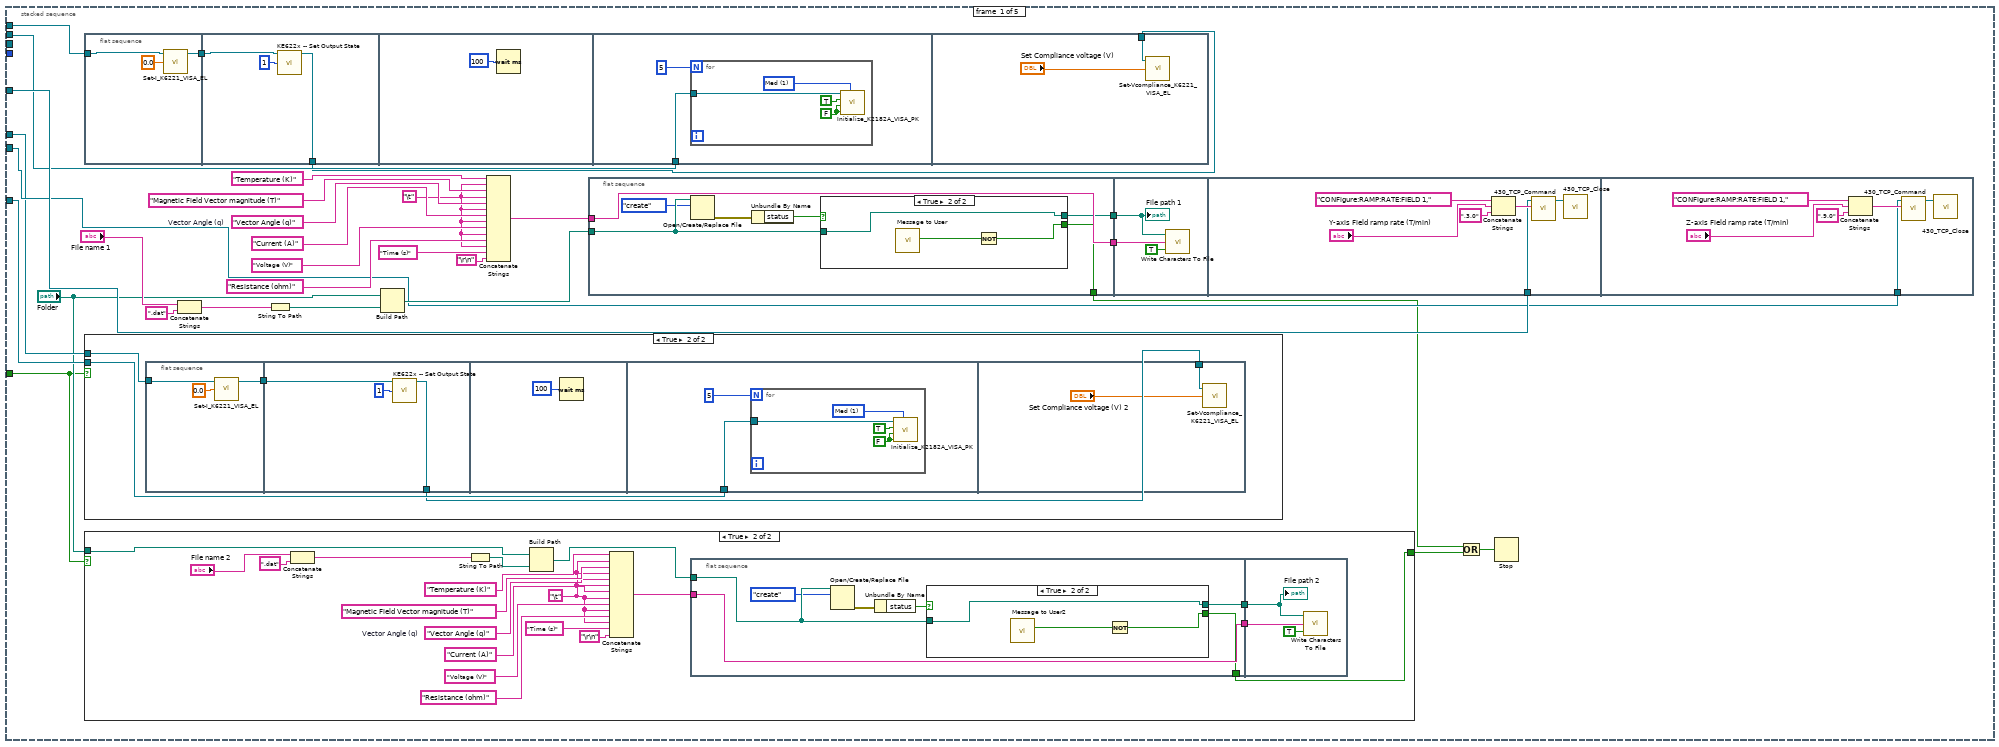
[diagram p2: hidden frame]
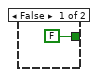
[diagram p3: hidden frame]
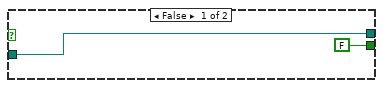
[diagram p4: hidden frame]
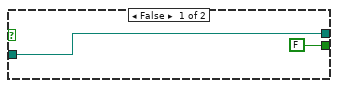
[diagram p6: hidden frame]
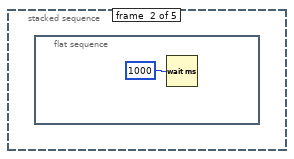
[diagram p7: hidden frame]
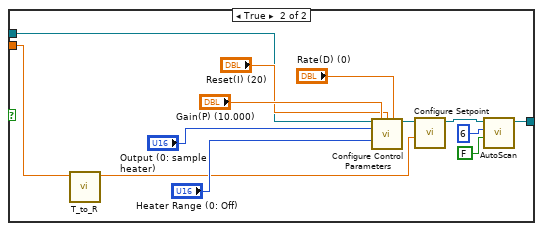
[diagram p9: hidden frame]
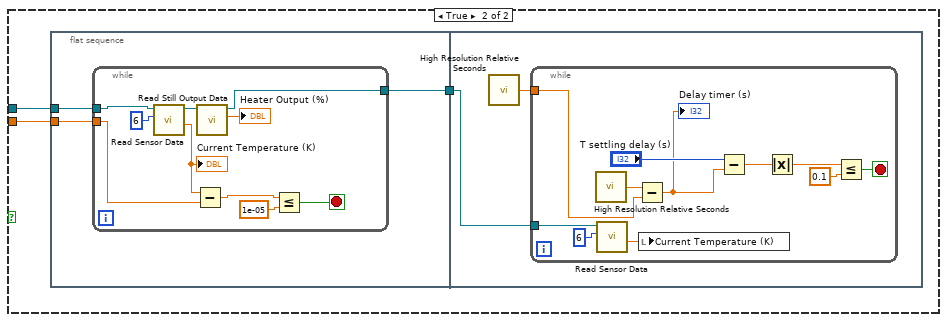
[diagram p10: hidden frame]
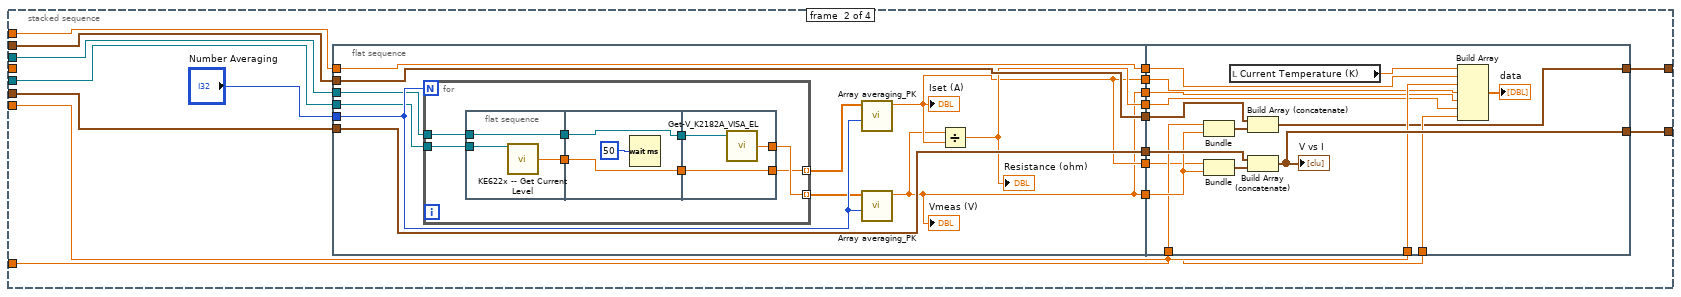
[diagram p13: hidden frame]
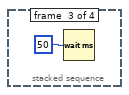
[diagram p14: hidden frame]
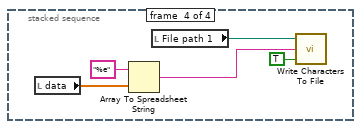
[diagram p15: hidden frame]
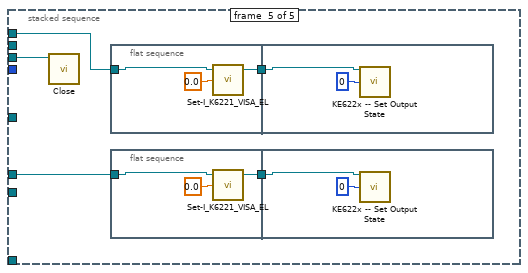
[diagram p16: hidden frame]
diagram:
  n1 = call "430_TCP_Open.vi"("IP Address"="Magnet IP Address Y-axis", "TCP Port"=7180) -> ("connection ID"=w12:refnum<k5>)  [unwired: 4 in, 2 out]
  n2 = call "430_TCP_Open.vi"("IP Address"="Magnet IP Address Z-axis", "TCP Port"=7180) -> ("connection ID"=w7:refnum<k5>)  [unwired: 4 in, 2 out]
  n3 = Tick Count (ms)() -> (millisecond timer value=w11:u32)
  n4 = stacked-sequence {
    tunnel: w12 -> [w31 _ _ _ _]
    tunnel: w11 -> [_ _ _ w166 _]
    tunnel: w7 -> [w28 _ _ _ _]
    tunnel: "Current source K6221 VISA Device 1" -> [w25 _ _ _ w628]
    tunnel: "Nanovoltmeter 2182a VISA Device1" -> [w24 _ _ _ _]
    tunnel: "Current source K6221 VISA Device 2" -> [w22 _ _ _ w626]
    tunnel: "Nanovoltmeter 2182a VISA Device 2" -> [w21 _ _ _ _]
    tunnel: "Measure two devices?" -> [w16 _ _ _ _]
    tunnel: refnum<visa-resource-name> "COM3" ("GPIB Mercury ITC") -> [_ _ _ w151 w625]
    frame #0 {
      w27 = "Vector Angle (q)"  # Vector Angle (q)
      w15 = "\t"
      n5 = flat-sequence {
        tunnel: w25 -> [w100]
        tunnel: [w98] -> w26
        tunnel: w26 -> [w103]
        tunnel: [w101] -> w23
        tunnel: w24 -> [w105]
        tunnel: w23 -> [w111]
        frame #0 {
          n6 = call "Set-I_K6221_VISA_EL.vi"("Set I (A)"=0.0, "K6221 VISA"=w100) -> ("K6221 VISA out"=w98:refnum<visa-resource-name>)  [unwired: 2 in, 1 out]
        }
        frame #1 {
          n7 = call "KE622x -- Set Output State.vi"("Resource In"=w103, "Output State"=1) -> ("Resource Out (dupl)"=w101:refnum<visa-resource-name>)  [unwired: 12 in, 1 out]
        }
        frame #2 {
          n8 = Wait (ms)(milliseconds to wait=100) -> ()  [unwired: 1 out]
        }
        frame #3 {
          n9 = for {
            N: 5 ("Numeric") -> [_]
            tunnel: w105 -> [w107]
            w109 = u16 1 items=["Slow", "Med", "Fast"] ("Rate (NPLC)")
            w110 = FALSE ("Auto range?")
            n10 = call "Initialize_K2182A_VISA_PK.vi"("VISA address"=w107, "Auto range?"=TRUE, "Analog LPass\nFilter?"=w110, "DC\nFilter?"=w110, "Rate (NPLC)"=w109) -> ()  [unwired: 2 in]
          }
        }
        frame #4 {
          n11 = call "Set-Vcompliance_K6221_VISA_EL.vi"("Set Compliance voltage (V)"="Set Compliance voltage (V)", "K6221 VISA"=w111) -> ()  [unwired: 2 in, 2 out]
        }
      }
      n12 = case shown="True" w16 {
        tunnel: w22 -> [_ w81]
        tunnel: w21 -> [_ w80]
        frame False {
        }
        frame True {
          n13 = flat-sequence {
            tunnel: w81 -> [w85]
            tunnel: [w83] -> w82
            tunnel: w82 -> [w88]
            tunnel: [w86] -> w79
            tunnel: w80 -> [w90]
            tunnel: w79 -> [w96]
            frame #0 {
              n14 = call "Set-I_K6221_VISA_EL.vi"("Set I (A)"=0.0, "K6221 VISA"=w85) -> ("K6221 VISA out"=w83:refnum<visa-resource-name>)  [unwired: 2 in, 1 out]
            }
            frame #1 {
              n15 = call "KE622x -- Set Output State.vi"("Resource In"=w88, "Output State"=1) -> ("Resource Out (dupl)"=w86:refnum<visa-resource-name>)  [unwired: 12 in, 1 out]
            }
            frame #2 {
              n16 = Wait (ms)(milliseconds to wait=100) -> ()  [unwired: 1 out]
            }
            frame #3 {
              n17 = for {
                N: 5 ("Numeric") -> [_]
                tunnel: w90 -> [w92]
                w94 = u16 1 items=["Slow", "Med", "Fast"] ("Rate (NPLC)")
                w95 = FALSE ("Auto range?")
                n18 = call "Initialize_K2182A_VISA_PK.vi"("VISA address"=w92, "Auto range?"=TRUE, "Analog LPass\nFilter?"=w95, "DC\nFilter?"=w95, "Rate (NPLC)"=w94) -> ()  [unwired: 2 in]
              }
            }
            frame #4 {
              n19 = call "Set-Vcompliance_K6221_VISA_EL.vi"("Set Compliance voltage (V)"="Set Compliance voltage (V) 2", "K6221 VISA"=w96) -> ()  [unwired: 2 in, 2 out]
            }
          }
        }
      }
      n20 = case shown="True" w16 {
        tunnel: [FALSE w48] -> w19
        tunnel: "Folder" -> [_ w47]
        frame False {
        }
        frame True {
          w49 = "Vector Angle (q)"  # Vector Angle (q)
          w46 = "\t"
          n21 = Concatenate Strings("File name 2", ".dat" ("string")) -> (w59:string)
          n22 = String To Path(string=w59) -> (path=w53:path)
          n23 = Build Path(base path=w47, name or relative path=w53) -> (appended path=w52:path)
          n24 = Concatenate Strings("Temperature (K)", w46, "Magnetic Field Vector magnitude (T)", w46, w49, w46, "Current (A)" ("string"), w46, "Voltage (V)" ("string"), w46, "Resistance (ohm)" ("string"), w46, "Time (s)", "\r\n") -> (w60:string)
          n25 = flat-sequence {
            tunnel: w52 -> [w68]
            tunnel: w60 -> [w70]
            tunnel: [w70] -> w62
            tunnel: [w69] -> w63
            tunnel: [w64] -> w48
            tunnel: w63 -> [w76]
            tunnel: w62 -> [w77]
            frame #0 {
              n26 = Open/Create/Replace File(file path (use dialog)=w68, operation (0:open)=T1."create") -> (error out=w67:errorcluster)  [unwired: 4 in, 2 out]
              n27 = Unbundle By Name(w67) -> ("status"=w65:bool)
              n28 = case shown="True" w65 {
                tunnel: [FALSE ("Yes") w74] -> w64
                tunnel: [w71 w73] -> w69
                tunnel: w68 -> [w71 w73]
                frame False {
                }
                frame True {
                  n29 = call "Message to User2"() -> ("Yes"=w75:bool)  [unwired: 10 in, 1 out]
                  n30 = Not(x=w75) -> (.not. x?=w74:bool)
                }
              }
            }
            frame #1 {
              n31 = call <vilib>:"Write Characters To File.vi"("append to file? (new file:F)"=TRUE, "character string"=w77, "file path (dialog if empty)"=w76) -> ()  [unwired: 2 in, 1 out]
              "File path 2" <- w76
            }
          }
        }
      }
      n32 = Concatenate Strings("File name 1", ".dat" ("string")) -> (w39:string)
      n33 = String To Path(string=w39) -> (path=w33:path)
      n34 = Build Path(base path="Folder", name or relative path=w33) -> (appended path=w32:path)
      n35 = Concatenate Strings("Temperature (K)", w15, "Magnetic Field Vector magnitude (T)", w15, w27, w15, "Current (A)" ("string"), w15, "Voltage (V)" ("string"), w15, "Resistance (ohm)" ("string"), w15, "Time (s)", "\r\n") -> (w40:string)
      n36 = flat-sequence {
        tunnel: w32 -> [w116]
        tunnel: w40 -> [w119]
        tunnel: [w119] -> w43
        tunnel: [w118] -> w20
        tunnel: [w117] -> w42
        tunnel: w43 -> [w126]
        tunnel: w42 -> [w125]
        tunnel: w31 -> [w129]
        tunnel: w28 -> [w134]
        frame #0 {
          n37 = Open/Create/Replace File(file path (use dialog)=w116, operation (0:open)=T1."create") -> (error out=w115:errorcluster)  [unwired: 4 in, 2 out]
          n38 = Unbundle By Name(w115) -> ("status"=w113:bool)
          n39 = case shown="True" w113 {
            tunnel: [FALSE ("Yes") w123] -> w118
            tunnel: [w120 w122] -> w117
            tunnel: w116 -> [w120 w122]
            frame False {
            }
            frame True {
              n40 = call "Message to User"() -> ("Yes"=w124:bool)  [unwired: 10 in, 1 out]
              n41 = Not(x=w124) -> (.not. x?=w123:bool)
            }
          }
        }
        frame #1 {
          n42 = call <vilib>:"Write Characters To File.vi"("append to file? (new file:F)"=TRUE, "character string"=w126, "file path (dialog if empty)"=w125) -> ()  [unwired: 2 in, 1 out]
          "File path 1" <- w125
        }
        frame #2 {
          n43 = Concatenate Strings("CONFigure:RAMP:RATE:FIELD 1," ("String"), "Y-axis Field ramp rate (T/min)", ",3.0") -> (w130:string)
          n44 = call "430_TCP_Command.vi"("Command"=w130, "connection ID"=w129) -> ("connection ID out"=w133:refnum<k5>)  [unwired: 2 in, 2 out]
          n45 = call "430_TCP_Close.vi"("connection ID"=w133) -> ()  [unwired: 1 in, 2 out]
        }
        frame #3 {
          n46 = Concatenate Strings("CONFigure:RAMP:RATE:FIELD 1," ("String"), "Z-axis Field ramp rate (T/min)", ",9.0") -> (w136:string)
          n47 = call "430_TCP_Command.vi"("Command"=w136, "connection ID"=w134) -> ("connection ID out"=w139:refnum<k5>)  [unwired: 2 in, 2 out]
          n48 = call "430_TCP_Close.vi"("connection ID"=w139) -> ()  [unwired: 1 in, 2 out]
        }
      }
      n49 = Or(x=w20, y=w19) -> (x .or. y?=w18:bool)
      n50 = Stop(stop? (T)=w18) -> ()
    }
    frame #1 {
      n51 = flat-sequence {
        frame #0 {
          n52 = Wait (ms)(milliseconds to wait=u32 1000) -> ()  [unwired: 1 out]
        }
      }
    }
    frame #2 {
    }
    frame #3 {
      w145 = u16 1 items=["Off", "31.6 uA", "100 uA", "316 uA", "1.00 mA", "3.16 mA", "10.0 mA", "31.6 mA", "100 mA"] ("Heater Range (0: Off)")
      w146 = u16 2 items=["sample heater", "output 1 (warm-up heater) ", "output 2 (analog/still)"] ("Output (0: sample heater)")
      w155 = u16 0 items=["sample heater", "output 1 (warm-up heater) ", "output 2 (analog/still)"] ("Output (0: sample heater)")
      w154 = u16 0 items=["Unipolar", "Bipolar"] ("Polarity (0: Unipolar)")
      w153 = u16 5 items=["Off", "Monitor Out", "Open Loop (Manual)", "Zone", "Still", "Closed Loop (PID)", "Warm-up"] ("Output Mode (0: Off)")
      w152 = u16 6 items=["1"=1, "2"=2, "3"=3, "4"=4, "5"=5, "6"=6, "7"=7, "8"=8, "9"=9, "10"=10, "11"=11, "12"=12, "13"=13, "14"=14, "15"=15, "16"=16, "A (Control Input)"=17] ("Channel (1:1)")
      w159 = u16 0 items=["none", "1", "2", "3", "4", "5", "6", "7", "8", "9", "10", "11", "12", "13", "14", "15", "16", "A (Control Input)"] ("Channel (1:1)")
      w161 = u16 4 items=["Off"=0, "Monitor Out"=1, "Open Loop (Manual)"=2, "Still"=4] ("Analog Out Mode (0: Off)")
      w162 = u16 2 items=["Kelvin"=1, "Ohms"=2] ("Source (1: Kelvin)")
      n53 = call "Initialize.vi"("Reset (True)"=FALSE, "ID Query (True)"=TRUE, "VISA resource name"=w151) -> ("VISA resource name out"=w156:refnum<visa-resource-name>)  [unwired: 7 in, 1 out]
      n54 = call "Configure Analog Still Output.vi"("VISA resource name"=w156, "Analog Out Mode (0: Off)"=w161, "Source (1: Kelvin)"=w162, "Enable Bipolar Mode (F: Disable)"=FALSE, "Channel (1:1)"=w159, "High Value (0.00000E+0)"=0.0, "Low Value (0.00000E+0)"=0.0, "Manual Value (0.000%)"=0.0, "Still Value (0.000%)"="Still Heater Output (%)") -> ("VISA resource name out"=w143:refnum<visa-resource-name>)  [unwired: 5 in, 1 out]
      n55 = call "Configure Control Parameters.vi"("VISA resource name"=w143, "Output (0: sample heater)"=w146, "Manual Output (0.000%)"=0.0, "Heater Range (0: Off)"=w145) -> ("VISA resource name out"=w142:refnum<visa-resource-name>)  [unwired: 10 in, 1 out]
      n56 = call "Configure Control Mode.vi"("VISA resource name"=w142, "Output (0: sample heater)"=w155, "Channel (1:1)"=w152, "Output Mode (0: Off)"=w153, "Polarity (0: Unipolar)"=w154) -> ("VISA resource name out"=w150:refnum<visa-resource-name>)  [unwired: 9 in, 1 out]
      n57 = for {
        tunnel: w166 -> [w184]
        tunnel: w150 -> [w172]
        tunnel: "From 5" -> [w182] mode=indexing
        tunnel: "Step 5" -> [w181] mode=indexing
        tunnel: "To 5" -> [w180] mode=indexing
        shift-right: [w170] -> _
        shift-left: "Still Heater Output (%)" -> [w171]
        w175 = u16 0 items=["none", "1", "2", "3", "4", "5", "6", "7", "8", "9", "10", "11", "12", "13", "14", "15", "16", "A (Control Input)"] ("Channel (1:1)")
        w177 = u16 4 items=["Off"=0, "Monitor Out"=1, "Open Loop (Manual)"=2, "Still"=4] ("Analog Out Mode (0: Off)")
        w178 = u16 2 items=["Kelvin"=1, "Ohms"=2] ("Source (1: Kelvin)")
        n58 = call "Build_serie_EL.vi"("end value"=w180, "increment"=w181, "start value"=w182) -> ("output array"=w183:dbl[])
        n59 = call "Configure Analog Still Output.vi"("VISA resource name"=w172, "Analog Out Mode (0: Off)"=w177, "Source (1: Kelvin)"=w178, "Enable Bipolar Mode (F: Disable)"=FALSE, "Channel (1:1)"=w175, "High Value (0.00000E+0)"=0.0, "Low Value (0.00000E+0)"=0.0, "Manual Value (0.000%)"=0.0, "Still Value (0.000%)"=w171) -> ("VISA resource name out"=w168:refnum<visa-resource-name>)  [unwired: 5 in, 1 out]
        n60 = call "Read Still Output Data.vi"("VISA resource name"=w168) -> ("Heater Output"=→"Still Output (%)":dbl, "VISA resource name out"=w167:refnum<visa-resource-name>)  [unwired: 8 in, 1 out]
        n61 = for {
          tunnel: w184 -> [w190]
          tunnel: w183 -> [w189] mode=indexing
          tunnel: w167 -> [w188]
          n62 = flat-sequence {
            tunnel: w190 -> [w198]
            tunnel: [w198] -> w192
            tunnel: w189 -> [w195]
            tunnel: w188 -> [w197]
            tunnel: [w196] -> w187
            tunnel: [w195] -> w186
            tunnel: [w193] -> w185
            tunnel: [w220] -> w191
            tunnel: w192 -> [w220]
            tunnel: w187 -> [w219]
            tunnel: w186 -> [w218]
            tunnel: w185 -> [w217]
            tunnel: w191 -> [w266]
            frame #0 {
              n63 = Greater?(x=w195, y=0.0) -> (0:w193:bool)
              n64 = case shown="False" w193 {
                tunnel: w197 -> [w203 w209]
                tunnel: w195 -> [_ w208]
                tunnel: [w202 w205] -> w196
                frame False {
                  w200 = u16 0 items=["Off", "31.6 uA", "100 uA", "316 uA", "1.00 mA", "3.16 mA", "10.0 mA", "31.6 mA", "100 mA"] ("Heater Range (0: Off)")
                  w201 = u16 0 items=["sample heater", "output 1 (warm-up heater) ", "output 2 (analog/still)"] ("Output (0: sample heater)")
                  n65 = call "Configure Control Parameters.vi"("VISA resource name"=w203, "Output (0: sample heater)"=w201, "Manual Output (0.000%)"=0.0, "Heater Range (0: Off)"=w200) -> ("VISA resource name out"=w202:refnum<visa-resource-name>)  [unwired: 10 in, 1 out]
                }
                frame True {
                  n66 = call "T_to_R.vi"("T to convert, K"=w208) -> ("R to set, Ohms"=w211:dbl)  [unwired: 9 in, 1 out]
                  n67 = call "Configure Control Parameters.vi"("VISA resource name"=w209, "Gain(P) (10.000)"="Gain(P) (10.000)", "Reset(I) (20)"="Reset(I) (20)", "Rate(D) (0)"="Rate(D) (0)", "Output (0: sample heater)"="Output (0: sample heater)", "Heater Range (0: Off)"="Heater Range (0: Off)") -> ("VISA resource name out"=w210:refnum<visa-resource-name>)  [unwired: 8 in, 1 out]
                  n68 = call "Configure Setpoint.vi"("Setpoint (0.00000E+0)"=w211, "VISA resource name"=w210) -> ("VISA resource name out"=w204:refnum<visa-resource-name>)  [unwired: 8 in, 1 out]
                  n69 = call "AutoScan.vi"("Autoscan (F: Off)"=FALSE, "Channel (1:1)"=6, "VISA resource name"=w204) -> ("VISA resource name out"=w205:refnum<visa-resource-name>)  [unwired: 7 in, 1 out]
                }
              }
              "Set Temperature (K)" <- w195
            }
            frame #1 {
              n70 = case shown="False" w217 {
                tunnel: w219 -> [w221 w235]
                tunnel: w218 -> [_ w234]
                frame False {
                  n71 = call <vilib>:"High Resolution Relative Seconds.vi"() -> ("relative seconds"=w222:dbl)
                  n72 = while {
                    tunnel: w222 -> [w232]
                    tunnel: w221 -> [w226]
                    stop <- w229 stop-if-true
                    n73 = call <vilib>:"High Resolution Relative Seconds.vi"() -> ("relative seconds"=w233:dbl)
                    n74 = call "Read Sensor Data.vi"("Channel (1:1)"=6, "VISA resource name"=w226) -> ("Kelvin Reading"=w225:dbl)  [unwired: 4 in, 5 out]
                    n75 = local read "T settling delay (s)"() -> (w224:i32)
                    n76 = Subtract(x=w233, y=w232) -> (x-y=w223:dbl)
                    n77 = local write "Current Temperature (K)"(w225) -> ()
                    n78 = local write "Delay timer (s)"(w223) -> ()
                    n79 = Subtract(x=w224, y=w223) -> (x-y=w231:dbl)
                    n80 = Absolute Value(x=w231) -> (abs(x)=w230:dbl)
                    n81 = Less Or Equal?(x=w230, y=0.1) -> (x <= y?=w229:bool)
                  }
                }
                frame True {
                  n82 = flat-sequence {
                    tunnel: w234 -> [w239]
                    tunnel: w235 -> [w238]
                    tunnel: [w237] -> w236
                    tunnel: w236 -> [w250]
                    frame #0 {
                      n83 = while {
                        tunnel: w239 -> [w245]
                        tunnel: w238 -> [w244]
                        tunnel: [w240] -> w237
                        stop <- w247 stop-if-true
                        n84 = call "Read Sensor Data.vi"("Channel (1:1)"=6, "VISA resource name"=w244) -> ("Kelvin Reading"=w241:dbl, "VISA resource name out"=w243:refnum<visa-resource-name>)  [unwired: 4 in, 4 out]
                        "Current Temperature (K)" <- w241
                        n85 = Subtract(x=w241, y=w245) -> (x-y=w246:dbl)
                        n86 = call "Read Still Output Data.vi"("VISA resource name"=w243) -> ("Heater Output"=→"Heater Output (%)":dbl, "VISA resource name out"=w240:refnum<visa-resource-name>)  [unwired: 8 in, 1 out]
                        n87 = Less Or Equal?(x=w246, y=1e-05) -> (x <= y?=w247:bool)
                      }
                    }
                    frame #1 {
                      n88 = call <vilib>:"High Resolution Relative Seconds.vi"() -> ("relative seconds"=w251:dbl)
                      n89 = while {
                        tunnel: w251 -> [w261]
                        tunnel: w250 -> [w253]
                        stop <- w256 stop-if-true
                        n90 = call <vilib>:"High Resolution Relative Seconds.vi"() -> ("relative seconds"=w262:dbl)
                        n91 = call "Read Sensor Data.vi"("Channel (1:1)"=6, "VISA resource name"=w253) -> ("Kelvin Reading"=w252:dbl)  [unwired: 4 in, 5 out]
                        n92 = Subtract(x=w262, y=w261) -> (x-y=w259:dbl)
                        "Delay timer (s)" <- w259
                        n93 = local write "Current Temperature (K)"(w252) -> ()
                        n94 = Subtract(x="T settling delay (s)", y=w259) -> (x-y=w258:dbl)
                        n95 = Absolute Value(x=w258) -> (abs(x)=w257:dbl)
                        n96 = Less Or Equal?(x=w257, y=0.1) -> (x <= y?=w256:bool)
                      }
                    }
                  }
                }
              }
            }
            frame #2 {
              n97 = for {
                tunnel: w266 -> [w271]
                tunnel: "From 2" -> [w270] mode=indexing
                tunnel: "To 2" -> [w269] mode=indexing
                tunnel: "Step 2" -> [w268] mode=indexing
                n98 = call "Build_serie_EL.vi"("end value"=w269, "increment"=w268, "start value"=w270) -> ("output array"=w267:dbl[])
                n99 = for {
                  tunnel: w271 -> [w273]
                  tunnel: w267 -> [w272] mode=indexing
                  n100 = for {
                    tunnel: "From" -> [w286] mode=indexing
                    tunnel: "To" -> [w284] mode=indexing
                    tunnel: "Step" -> [w285] mode=indexing
                    tunnel: w273 -> [w283]
                    tunnel: w272 -> [w278]
                    n101 = flat-sequence {
                      tunnel: w283 -> [w288]
                      tunnel: w284 -> [w289]
                      tunnel: w285 -> [w290]
                      tunnel: w286 -> [w291]
                      tunnel: [w291] -> w282
                      tunnel: [w290] -> w281
                      tunnel: [w289] -> w280
                      tunnel: [w288] -> w279
                      tunnel: w278 -> [w287]
                      tunnel: [w287] -> w277
                      tunnel: w282 -> [w297]
                      tunnel: w281 -> [w296]
                      tunnel: w280 -> [w295]
                      tunnel: w279 -> [w293]
                      tunnel: w277 -> [w292]
                      frame #0 {
                      }
                      frame #1 {
                        n102 = call "Build_serie_EL.vi"("end value"=w295, "increment"=w296, "start value"=w297) -> ("output array"=w294:dbl[])
                        n103 = for {
                          tunnel: w294 -> [w311] mode=indexing
                          tunnel: w293 -> [w310]
                          tunnel: w292 -> [w309]
                          n104 = flat-sequence {
                            tunnel: [w314] -> w308
                            tunnel: [w315] -> w307
                            tunnel: w309 -> [w312]
                            tunnel: w311 -> [w313]
                            tunnel: w308 -> [w332]
                            tunnel: [w332] -> w304
                            tunnel: [w331] -> w306
                            tunnel: w307 -> [w331]
                            tunnel: [w330] -> w302
                            tunnel: [w329] -> w301
                            tunnel: [w328] -> w300
                            tunnel: [w327] -> w299
                            tunnel: w306 -> [w350]
                            tunnel: [w350] -> w305
                            tunnel: w304 -> [w349]
                            tunnel: [w349] -> w303
                            tunnel: w302 -> [w344]
                            tunnel: w301 -> [w343]
                            tunnel: w300 -> [w342]
                            tunnel: w299 -> [w341]
                            tunnel: [w340] -> w298
                            tunnel: w305 -> [w426]
                            tunnel: w303 -> [w420]
                            tunnel: w310 -> [w427]
                            tunnel: w298 -> [w414]
                            frame #0 {
                              n105 = local read "Z-axis Field ramp rate (T/min)"() -> (w323:string)
                              n106 = local read "Y-axis Field ramp rate (T/min)"() -> (w324:string)
                              n107 = local read "Magnet IP Address Z-axis"() -> (w326:string)
                              n108 = local read "Magnet IP Address Y-axis"() -> (w325:string)
                              n109 = call "Set2D_Magneticfield(polar)_PK.vi"("Y-axis Ramp Rate (T/min)"=w324, "Z-axis Ramp Rate (T/min)"=w323, "Set target vector angle (degrees)"=w313, "Set target vector magnitude (T)"=w312, "Y-Axis Magnet IP Address"=w325, "Z-Axis Magnet IP Address"=w326) -> ("Z-axis Magnetic Field (T)"=w320:string, "Y-axis Magnetic Field (T)"=w322:string, "q - Vector angle"=w315:dbl, "R - Vector field magnitude (T)"=w314:dbl)  [unwired: 2 in]
                              "Z-axis Magnetic Field (T)" <- w320
                              "Y-axis Magnetic Field (T)" <- w322
                              "Magnetic Field Vector magnitude (T)" <- w314
                              "Magnetic Field Vector Angle" <- w315
                              n110 = Build Array(w315) -> (w316:dbl[])
                              n111 = Build Array(w314) -> (w317:dbl[])
                              n112 = Fract/Exp String To Number(string=w322) -> (number=→"Y-Axis (0deg)":dbl)  [unwired: 3 in, 1 out]
                              n113 = Fract/Exp String To Number(string=w320) -> (number=→"Z-axis (90 deg)":dbl)  [unwired: 3 in, 1 out]
                              n114 = call-poly <vilib>:"Plot Helper.vi"("radius vector"=w317, "theta vector"=w316) -> ("2D Plot Class Obj Array out"=→"2D Compass":refnum<class "2D Plot Datatype.lvclass">[])  [unwired: 2 in, 7 out]
                            }
                            frame #1 {
                              n115 = local read "Nanovoltmeter 2182a VISA Device 2"() -> (w327:refnum<visa-resource-name>)
                              n116 = local read "Current source K6221 VISA Device 1"() -> (w330:refnum<visa-resource-name>)
                              n117 = local read "Current source K6221 VISA Device 2"() -> (w328:refnum<visa-resource-name>)
                              n118 = local read "Nanovoltmeter 2182a VISA Device1"() -> (w329:refnum<visa-resource-name>)
                              n119 = Multiply(x="Magnetic field stabilization time (s)", y=1000) -> (x*y=w334:dbl)
                              n120 = Wait (ms)(milliseconds to wait=w334) -> ()  [unwired: 1 out]
                            }
                            frame #2 {
                              n121 = flat-sequence {
                                tunnel: w344 -> [w399]
                                tunnel: [w397] -> w348
                                tunnel: w348 -> [w402]
                                tunnel: [w400] -> w347
                                tunnel: w347 -> [w403]
                                tunnel: [w403] -> w346
                                tunnel: w346 -> [w406]
                                tunnel: [w406] -> w345
                                tunnel: w343 -> [w405]
                                tunnel: w345 -> [w412]
                                frame #0 {
                                n122 = call "Set-I_K6221_VISA_EL.vi"("Set I (A)"=0.0, "K6221 VISA"=w399) -> ("K6221 VISA out"=w397:refnum<visa-resource-name>)  [unwired: 2 in, 1 out]
                                }
                                frame #1 {
                                n123 = call "KE622x -- Set Output State.vi"("Resource In"=w402, "Output State"=1) -> ("Resource Out (dupl)"=w400:refnum<visa-resource-name>)  [unwired: 12 in, 1 out]
                                }
                                frame #2 {
                                n124 = Wait (ms)(milliseconds to wait=100) -> ()  [unwired: 1 out]
                                }
                                frame #3 {
                                n125 = for {
                                N: 5 ("Numeric") -> [_]
                                tunnel: w405 -> [w408]
                                w410 = u16 1 items=["Slow", "Med", "Fast"] ("Rate (NPLC)")
                                w411 = FALSE ("Auto range?")
                                n126 = call "Initialize_K2182A_VISA_PK.vi"("VISA address"=w408, "Auto range?"=TRUE, "Analog LPass\nFilter?"=w411, "DC\nFilter?"=w411, "Rate (NPLC)"=w410) -> ()  [unwired: 2 in]
                                }
                                }
                                frame #4 {
                                n127 = local read "Set Compliance voltage (V)"() -> (w413:dbl)
                                n128 = call "Set-Vcompliance_K6221_VISA_EL.vi"("Set Compliance voltage (V)"=w413, "K6221 VISA"=w412) -> ()  [unwired: 2 in, 2 out]
                                }
                              }
                              n129 = local read "Measure two devices?"() -> (w340:bool)
                              n130 = flat-sequence {
                                tunnel: refnum<visa-resource-name> "COM3" ("VISA resource name") -> [w353]
                                tunnel: [w356] -> w339
                                tunnel: w339 -> [w359]
                                tunnel: [w363] -> w338
                                tunnel: w338 -> [w366]
                                tunnel: [w365] -> w336
                                tunnel: w336 -> [w369]
                                frame #0 {
                                n131 = call "AutoScan.vi"("Autoscan (F: Off)"=FALSE, "Channel (1:1)"=3, "VISA resource name"=w353) -> ("VISA resource name out"=w351:refnum<visa-resource-name>)  [unwired: 7 in, 1 out]
                                n132 = call "Read Sensor Data.vi"("Channel (1:1)"=3, "VISA resource name"=w351) -> ("Kelvin Reading"=→"Magnet temperature (K)":dbl, "VISA resource name out"=w356:refnum<visa-resource-name>)  [unwired: 4 in, 4 out]
                                }
                                frame #1 {
                                n133 = call "AutoScan.vi"("Autoscan (F: Off)"=FALSE, "Channel (1:1)"=6, "VISA resource name"=w359) -> ("VISA resource name out"=w358:refnum<visa-resource-name>)  [unwired: 7 in, 1 out]
                                n134 = call "Read Sensor Data.vi"("Channel (1:1)"=6, "VISA resource name"=w358) -> ("Kelvin Reading"=w362:dbl, "VISA resource name out"=w363:refnum<visa-resource-name>)  [unwired: 4 in, 4 out]
                                n135 = local write "Current Temperature (K)"(w362) -> ()
                                }
                                frame #2 {
                                n136 = call "Read Still Output Data.vi"("VISA resource name"=w366) -> ("Heater Output"=w367:dbl, "VISA resource name out"=w365:refnum<visa-resource-name>)  [unwired: 8 in, 1 out]
                                n137 = local write "Heater Output (%)"(w367) -> ()
                                }
                                frame #3 {
                                n138 = call "AutoScan.vi"("Autoscan (F: Off)"=FALSE, "Channel (1:1)"=5, "VISA resource name"=w369) -> ("VISA resource name out"=w370:refnum<visa-resource-name>)  [unwired: 7 in, 1 out]
                                n139 = call "Read Sensor Data.vi"("Channel (1:1)"=5, "VISA resource name"=w370) -> ("Kelvin Reading"=→"Still temperature (K)":dbl)  [unwired: 4 in, 5 out]
                                }
                              }
                              n140 = case shown="True" w340 {
                                tunnel: w342 -> [_ w375]
                                tunnel: w341 -> [_ w374]
                                frame False {
                                }
                                frame True {
                                n141 = flat-sequence {
                                tunnel: w375 -> [w382]
                                tunnel: [w380] -> w379
                                tunnel: w379 -> [w385]
                                tunnel: [w383] -> w378
                                tunnel: w378 -> [w386]
                                tunnel: [w386] -> w377
                                tunnel: w377 -> [w389]
                                tunnel: [w389] -> w376
                                tunnel: w374 -> [w388]
                                tunnel: w376 -> [w395]
                                frame #0 {
                                n142 = call "Set-I_K6221_VISA_EL.vi"("Set I (A)"=0.0, "K6221 VISA"=w382) -> ("K6221 VISA out"=w380:refnum<visa-resource-name>)  [unwired: 2 in, 1 out]
                                }
                                frame #1 {
                                n143 = call "KE622x -- Set Output State.vi"("Resource In"=w385, "Output State"=1) -> ("Resource Out (dupl)"=w383:refnum<visa-resource-name>)  [unwired: 12 in, 1 out]
                                }
                                frame #2 {
                                n144 = Wait (ms)(milliseconds to wait=100) -> ()  [unwired: 1 out]
                                }
                                frame #3 {
                                n145 = for {
                                N: 5 ("Numeric") -> [_]
                                tunnel: w388 -> [w391]
                                w393 = u16 1 items=["Slow", "Med", "Fast"] ("Rate (NPLC)")
                                w394 = FALSE ("Auto range?")
                                n146 = call "Initialize_K2182A_VISA_PK.vi"("VISA address"=w391, "Auto range?"=TRUE, "Analog LPass\nFilter?"=w394, "DC\nFilter?"=w394, "Rate (NPLC)"=w393) -> ()  [unwired: 2 in]
                                }
                                }
                                frame #4 {
                                n147 = local read "Set Compliance voltage (V) 2"() -> (w396:dbl)
                                n148 = call "Set-Vcompliance_K6221_VISA_EL.vi"("Set Compliance voltage (V)"=w396, "K6221 VISA"=w395) -> ()  [unwired: 2 in, 2 out]
                                }
                                }
                                }
                              }
                            }
                            frame #3 {
                              n149 = for {
                                tunnel: w427 -> [w533]
                                tunnel: w420 -> [w531]
                                tunnel: w426 -> [w530]
                                tunnel: "From 3" -> [w525] mode=indexing
                                tunnel: "Step 3" -> [w524] mode=indexing
                                tunnel: "To 3" -> [w523] mode=indexing
                                shift-right: [w522] -> _
                                shift-left: cluster{dbl, "Field Reading":dbl}[] [] -> [w529]
                                shift-right: [w521] -> _
                                shift-left: cluster{dbl, "Field Reading":dbl}[] [] -> [w532]
                                n150 = call "Build_serie_EL.vi"("end value"=w523, "increment"=w524, "start value"=w525) -> ("output array"=w526:dbl[])
                                n151 = local read "Current source K6221 VISA Device 1"() -> (w528:refnum<visa-resource-name>)
                                n152 = local read "Nanovoltmeter 2182a VISA Device1"() -> (w527:refnum<visa-resource-name>)
                                n153 = for {
                                tunnel: w533 -> [w547]
                                tunnel: w531 -> [w541]
                                tunnel: w530 -> [w540]
                                tunnel: w526 -> [w538] mode=indexing
                                shift-right: [w534] -> w521
                                shift-left: w532 -> [w546]
                                shift-right: [w535] -> w522
                                shift-left: w529 -> [w539]
                                tunnel: w528 -> [w537]
                                tunnel: w527 -> [w536]
                                n154 = Tick Count (ms)() -> (millisecond timer value=w543:u32)
                                n155 = Subtract(x=w543, y=w547) -> (x-y=w545:u32)
                                n156 = Divide(x=w545, y=1000.0) -> (x/y=w542:dbl)
                                "Time (s)" <- w542
                                n157 = stacked-sequence {
                                tunnel: w546 -> [_ w569 _ _]
                                tunnel: [_ w570 _ _] -> w534
                                tunnel: w542 -> [_ w557 _ _]
                                tunnel: w541 -> [_ w564 _ _]
                                tunnel: w540 -> [_ w563 _ _]
                                tunnel: [_ w562 _ _] -> w535
                                tunnel: w539 -> [_ w560 _ _]
                                tunnel: w538 -> [w549 _ _ _]
                                tunnel: w537 -> [w548 w554 _ _]
                                tunnel: w536 -> [_ w553 _ _]
                                frame #0 {
                                n158 = flat-sequence {
                                tunnel: w549 -> [w551]
                                tunnel: w548 -> [w550]
                                frame #0 {
                                n159 = call "Set-I_K6221_VISA_EL.vi"("Set I (A)"=w551, "K6221 VISA"=w550) -> ()  [unwired: 2 in, 2 out]
                                }
                                frame #1 {
                                n160 = Wait (ms)(milliseconds to wait="wait (ms)") -> ()  [unwired: 1 out]
                                }
                                }
                                }
                                frame #1 {
                                n161 = flat-sequence {
                                tunnel: [w575] -> w568
                                tunnel: [w581] -> w567
                                tunnel: [w577] -> w566
                                tunnel: [w580] -> w565
                                tunnel: [w579] -> w561
                                tunnel: "Number Averaging" -> [w574]
                                tunnel: w560 -> [w579]
                                tunnel: w569 -> [w581]
                                tunnel: w564 -> [w580]
                                tunnel: [w575] -> w558
                                tunnel: [w577] -> w556
                                tunnel: [w578] -> w555
                                tunnel: w554 -> [w572]
                                tunnel: w553 -> [w571]
                                tunnel: w568 -> [w604]
                                tunnel: [w614] -> w570
                                tunnel: w567 -> [w613]
                                tunnel: w566 -> [w603]
                                tunnel: w565 -> [w608]
                                tunnel: w557 -> [w611]
                                tunnel: w563 -> [w610]
                                tunnel: [w606] -> w562
                                tunnel: w561 -> [w605]
                                tunnel: w558 -> [w607]
                                tunnel: w557 -> [w602]
                                tunnel: w556 -> [w601]
                                tunnel: w555 -> [w600]
                                frame #0 {
                                n162 = for {
                                N: w574 -> [_]
                                tunnel: [w583] -> w573 mode=indexing
                                tunnel: [w582] -> w576 mode=indexing
                                tunnel: w572 -> [w588]
                                tunnel: w571 -> [w589]
                                n163 = flat-sequence {
                                tunnel: w588 -> [w590]
                                tunnel: w589 -> [w592]
                                tunnel: [w592] -> w587
                                tunnel: [w591] -> w586
                                tunnel: w587 -> [w595]
                                tunnel: w586 -> [w594]
                                tunnel: [w595] -> w585
                                tunnel: [w594] -> w584
                                tunnel: [w598] -> w582
                                tunnel: w585 -> [w597]
                                tunnel: w584 -> [w598]
                                tunnel: [w596] -> w583
                                frame #0 {
                                n164 = call "KE622x -- Get Current Level.vi"("Resource In"=w590) -> ("Current Level (A)"=w591:T2)  [unwired: 12 in, 2 out]
                                }
                                frame #1 {
                                n165 = Wait (ms)(milliseconds to wait=50) -> ()  [unwired: 1 out]
                                }
                                frame #2 {
                                n166 = call "Get-V_K2182A_VISA_EL.vi"("VISA K2182A"=w597) -> ("V (V)"=w596:dbl)  [unwired: 2 in, 2 out]
                                }
                                }
                                }
                                n167 = call "Array averaging_PK.vi"("Number averaging"=w574, "numeric array"=w576) -> ("Average value"=w577:dbl)  [unwired: 9 in]
                                "Iset (A)" <- w577
                                n168 = call "Array averaging_PK.vi"("Number averaging"=w574, "numeric array"=w573) -> ("Average value"=w575:dbl)  [unwired: 9 in]
                                "Vmeas (V)" <- w575
                                n169 = Divide(x=w575, y=w577) -> (x/y=w578:dbl)
                                "Resistance (ohm)" <- w578
                                }
                                frame #1 {
                                n170 = Bundle(w602, "Average value"=w607) -> (w609:cluster{dbl, "Average value":dbl})  [unwired: 1 in]
                                n171 = Bundle("Average value"=w601, "Average value"=w607) -> (w612:T3)  [unwired: 1 in]
                                n172 = local read "Current Temperature (K)"() -> (w599:dbl)
                                n173 = Build Array (concatenate)(w605, w609) -> (w606:cluster{dbl, "Average value":dbl}[])
                                n174 = Build Array (concatenate)(w613, w612) -> (w614:T4)
                                "V vs I" <- w614
                                n175 = Build Array(w599, w608, w610, w603, w604, w600, w611) -> (→"data":dbl[])
                                }
                                }
                                }
                                frame #2 {
                                n176 = Wait (ms)(milliseconds to wait=u32 50) -> ()  [unwired: 1 out]
                                }
                                frame #3 {
                                n177 = local read "data"() -> (w617:dbl[])
                                n178 = Array To Spreadsheet String(array=w617, 3:"%e" ("format string")) -> (spreadsheet string=w620:string)  [unwired: 1 in]
                                n179 = local read "File path 1"() -> (w619:path)
                                n180 = call <vilib>:"Write Characters To File.vi"("append to file? (new file:F)"=TRUE, "character string"=w620, "file path (dialog if empty)"=w619) -> ()  [unwired: 2 in, 1 out]
                                }
                                }
                                }
                              }
                              n181 = case shown="True" w414 {
                                tunnel: "From 4" -> [_ w432]
                                tunnel: "To 4" -> [_ w431]
                                tunnel: "Step 4" -> [_ w430]
                                tunnel: cluster{dbl, "Field Reading":dbl}[] [] -> [_ w429]
                                tunnel: cluster{dbl, "Field Reading":dbl}[] [] -> [_ w428]
                                frame False {
                                }
                                frame True {
                                n182 = for {
                                tunnel: w432 -> [w439] mode=indexing
                                tunnel: w431 -> [w438] mode=indexing
                                tunnel: w430 -> [w437] mode=indexing
                                shift-right: [w434] -> _
                                shift-left: w429 -> [w436]
                                shift-right: [w433] -> _
                                shift-left: w428 -> [w435]
                                n183 = call "Build_serie_EL.vi"("end value"=w438, "increment"=w437, "start value"=w439) -> ("output array"=w440:dbl[])
                                n184 = local read "Nanovoltmeter 2182a VISA Device 2"() -> (w441:refnum<visa-resource-name>)
                                n185 = local read "Current source K6221 VISA Device 2"() -> (w442:refnum<visa-resource-name>)
                                n186 = for {
                                tunnel: w440 -> [w448] mode=indexing
                                shift-right: [w444] -> w433
                                shift-left: w435 -> [w450]
                                shift-right: [w445] -> w434
                                shift-left: w436 -> [w449]
                                tunnel: w442 -> [w447]
                                tunnel: w441 -> [w446]
                                n187 = local read "Time (s)"() -> (w443:dbl)
                                n188 = stacked-sequence {
                                tunnel: w450 -> [_ w469 _ _]
                                tunnel: [_ w470 _ _] -> w444
                                tunnel: w443 -> [_ w461 _ _]
                                tunnel: [_ w465 _ _] -> w445
                                tunnel: w449 -> [_ w463 _ _]
                                tunnel: w448 -> [w452 _ _ _]
                                tunnel: w447 -> [w451 w458 _ _]
                                tunnel: w446 -> [_ w457 _ _]
                                frame #0 {
                                n189 = flat-sequence {
                                tunnel: w452 -> [w454]
                                tunnel: w451 -> [w453]
                                frame #0 {
                                n190 = call "Set-I_K6221_VISA_EL.vi"("Set I (A)"=w454, "K6221 VISA"=w453) -> ()  [unwired: 2 in, 2 out]
                                }
                                frame #1 {
                                n191 = Wait (ms)(milliseconds to wait="wait (ms) 2") -> ()  [unwired: 1 out]
                                }
                                }
                                }
                                frame #1 {
                                n192 = local read "Number Averaging"() -> (w456:i32)
                                n193 = flat-sequence {
                                tunnel: [w475] -> w468
                                tunnel: [w480] -> w467
                                tunnel: [w477] -> w466
                                tunnel: [w479] -> w464
                                tunnel: w456 -> [w474]
                                tunnel: w463 -> [w479]
                                tunnel: w469 -> [w480]
                                tunnel: [w475] -> w462
                                tunnel: [w477] -> w460
                                tunnel: [w478] -> w459
                                tunnel: w458 -> [w472]
                                tunnel: w457 -> [w471]
                                tunnel: w468 -> [w505]
                                tunnel: [w513] -> w470
                                tunnel: w467 -> [w512]
                                tunnel: w466 -> [w504]
                                tunnel: w461 -> [w510]
                                tunnel: [w507] -> w465
                                tunnel: w464 -> [w506]
                                tunnel: w462 -> [w508]
                                tunnel: w461 -> [w503]
                                tunnel: w460 -> [w502]
                                tunnel: w459 -> [w501]
                                frame #0 {
                                n194 = for {
                                N: w474 -> [_]
                                tunnel: [w482] -> w473 mode=indexing
                                tunnel: [w481] -> w476 mode=indexing
                                tunnel: w472 -> [w487]
                                tunnel: w471 -> [w488]
                                n195 = flat-sequence {
                                tunnel: w487 -> [w489]
                                tunnel: w488 -> [w491]
                                tunnel: [w491] -> w486
                                tunnel: [w490] -> w485
                                tunnel: w486 -> [w494]
                                tunnel: w485 -> [w493]
                                tunnel: [w494] -> w484
                                tunnel: [w493] -> w483
                                tunnel: [w497] -> w481
                                tunnel: w484 -> [w496]
                                tunnel: w483 -> [w497]
                                tunnel: [w495] -> w482
                                frame #0 {
                                n196 = call "KE622x -- Get Current Level.vi"("Resource In"=w489) -> ("Current Level (A)"=w490:T2)  [unwired: 12 in, 2 out]
                                }
                                frame #1 {
                                n197 = Wait (ms)(milliseconds to wait=50) -> ()  [unwired: 1 out]
                                }
                                frame #2 {
                                n198 = call "Get-V_K2182A_VISA_EL.vi"("VISA K2182A"=w496) -> ("V (V)"=w495:dbl)  [unwired: 2 in, 2 out]
                                }
                                }
                                }
                                n199 = call "Array averaging_PK.vi"("Number averaging"=w474, "numeric array"=w473) -> ("Average value"=w475:dbl)  [unwired: 9 in]
                                "Vmeas (V) 2" <- w475
                                n200 = call "Array averaging_PK.vi"("Number averaging"=w474, "numeric array"=w476) -> ("Average value"=w477:dbl)  [unwired: 9 in]
                                "Iset (A) 2" <- w477
                                n201 = Divide(x=w475, y=w477) -> (x/y=w478:dbl)
                                "Resistance (ohm) 2" <- w478
                                }
                                frame #1 {
                                n202 = Bundle("Time (s)"=w503, "Average value"=w508) -> (w509:cluster{"Time (s)":dbl, "Average value":dbl})  [unwired: 1 in]
                                n203 = Bundle("Average value"=w502, "Average value"=w508) -> (w511:T3)  [unwired: 1 in]
                                n204 = Build Array (concatenate)(w506, w509) -> (w507:cluster{"Time (s)":dbl, "Average value":dbl}[])
                                n205 = Build Array (concatenate)(w512, w511) -> (w513:T4)
                                "V vs I 2" <- w513
                                n206 = local read "Magnetic Field Vector magnitude (T)"() -> (w500:dbl)
                                n207 = local read "Magnetic Field Vector Angle"() -> (w499:dbl)
                                n208 = local read "Current Temperature (K)"() -> (w498:dbl)
                                n209 = Build Array(w498, w500, w499, w504, w505, w501, w510) -> (→"data 2":dbl[])
                                }
                                }
                                }
                                frame #2 {
                                n210 = Wait (ms)(milliseconds to wait=u32 50) -> ()  [unwired: 1 out]
                                }
                                frame #3 {
                                n211 = local read "data 2"() -> (w516:dbl[])
                                n212 = local read "File path 2"() -> (w518:path)
                                n213 = Array To Spreadsheet String(array=w516, 3:"%e" ("format string")) -> (spreadsheet string=w519:string)  [unwired: 1 in]
                                n214 = call <vilib>:"Write Characters To File.vi"("append to file? (new file:F)"=TRUE, "character string"=w519, "file path (dialog if empty)"=w518) -> ()  [unwired: 2 in, 1 out]
                                }
                                }
                                }
                                }
                                }
                              }
                            }
                          }
                        }
                      }
                      frame #2 {
                        n215 = Multiply(x="Wait time after each sweep(min)", y=60000.0) -> (x*y=w624:dbl)
                        n216 = Wait (ms)(milliseconds to wait=w624) -> ()  [unwired: 1 out]
                      }
                    }
                  }
                }
              }
            }
          }
        }
        n217 = local read "Still Heater Output (%)"() -> (w170:dbl)
      }
    }
    frame #4 {
      n218 = call "Close.vi"("VISA resource name"=w625) -> ()  [unwired: 10 in, 1 out]
      n219 = flat-sequence {
        tunnel: w628 -> [w637]
        tunnel: [w635] -> w629
        tunnel: w629 -> [w639]
        frame #0 {
          n220 = call "Set-I_K6221_VISA_EL.vi"("Set I (A)"=0.0, "K6221 VISA"=w637) -> ("K6221 VISA out"=w635:refnum<visa-resource-name>)  [unwired: 2 in, 1 out]
        }
        frame #1 {
          n221 = call "KE622x -- Set Output State.vi"("Resource In"=w639, "Output State"=0) -> ()  [unwired: 12 in, 2 out]
        }
      }
      n222 = flat-sequence {
        tunnel: w626 -> [w632]
        tunnel: [w630] -> w627
        tunnel: w627 -> [w634]
        frame #0 {
          n223 = call "Set-I_K6221_VISA_EL.vi"("Set I (A)"=0.0, "K6221 VISA"=w632) -> ("K6221 VISA out"=w630:refnum<visa-resource-name>)  [unwired: 2 in, 1 out]
        }
        frame #1 {
          n224 = call "KE622x -- Set Output State.vi"("Resource In"=w634, "Output State"=0) -> ()  [unwired: 12 in, 2 out]
        }
      }
    }
  }
